vi "Argos.vi"(0 "PID 1 COM":refnum<visa-resource-name>="COM8", 1 "Setpoint\n START":bool, 2 "Write to File":bool, 3 "SP 1 input (°C)":dbl=20.0 min=0.0 max=1300.0, 4 "Intervall (s)":u32=1 max=600 format="%.2f", 5 "Write/\nRead":bool=TRUE, 6 "Delay (ms)":u32=500 min=100 max=600000, 7 "Auto Tune":bool, 9 "Standby":bool, 11 "Reset\nSTOPP":bool, 12 "ON":bool=TRUE caption="OFF", 13 "Get Values":bool, 15 "File Path":path) -> (8 "(°C)":dbl format="%#.3f", 14 "SP 1 is (°C)":dbl)   [LabVIEW 2010]
doc: "1. Verwendung\n\nDas Programm dient der Steuerung und Abfrage des Thermocontrollers I3252 und dem Auslesen von zwei VC 840 Messgeräten und einem Druckmessgerät Pfeiffer Single Gauge. \nDie Messgeräte werden Standardmäßig ausgelesen und erst nach Betätigung des Schalters \"Write to File\" in einer Textdatei abgespeichert. Das Eingabefeld \"Intervall\" legt den Abstand der Messpunkte fest.\nDer Setpoint für den Thermocontroller wird erst nach Betätigung des Tasters \"Setpoint START\" übernommen und angesteuert. Er wird ind den EEPROM des Gerätes geschrieben. Die Regelung kann mit Hilfe des Schalters \"Standby\" unterbrochen werden. Durch den Taster \"Reset STOPP\" kann der Setpoint aus dem EEPROM gelöscht werden.\nDie Eingabeflächen \"Constant\" und \"Thickness\" dienen der Berechnung des spezifischen Widerstands.\nDie Eingabeflächen \"User\" und \"Sample\" werden in den Header der Textdatei übernommen.\nDer Indikator \"File Path\" zeigt den aktuellen Speicherort der Textdatei an. Dieser wird nach ausschalten des Schalters \"Write to File\" gelöscht. Bei erneuten Schreiben muss ein neuer Speicherort gewählt werden. Bei Wahl desselben Speicherorts werden sämtliche bereits gespeicherte Daten gelöscht.\n\n\n2. Erläuterungen zum Blockdiagramm\n2.1 äußere Sequenz\nDie äußerte Sequenz besteht aus fünf Frames. Der erste dient der Initialisierung der Ports. Der zweite dient als Verzögerung um dem Programm genug Zeit zu geben die Ports zu öffnen. Jedoch senden die beiden VC 840 bereits Informationen an den Computer die in einem Puffer zwischengespeichert werden. Im dritten Frame wird dieser Puffer geleert. Somit kommt es zu keinem Framing Error. Desweiteren wird in diesem Frame die Startzeit der Messungen genommen. Im vierten Frame wird die eigentliche Messung und Verarbeitung der Daten durchgeführt. Die while-Schleife wird nur durch Auftreten eines Fehlers oder durch Betätigung des Stopbuttons auf dem Front Panel in der oberen linken Ecke unterbrochen. Im fünften und letzten Frame werden die Ports wieder geschlossen und beim Auftreten eines Fehlers wird das Programm automatisch gestoppt. Falls kein Fehler auftritt wird die Sequenz von vorne abgearbeitet.\n\n2.2 while-Schleife und innere Sequenz\n2.2.1 \"Event Structure\"\n2.2.1.1 Allgemein\nDer erste Frame beinhaltet ein \"Event Structure\". Dieser reagiert auf insgesamt elf verschiedene Ereignisse. Falls keines dieser Ereignisse auftreten sollte, warte die Struktur eine Millisekunde bevor die \"Event Structure\" verlassen wird. Die übrigen Ereignisse treten ein, wenn der entsprechende Kontroller eine Werteänderung erfährt.\n\n2.2.1.2 Event: Setpoint\nDieser Case besteht von außen nach innen aus einer Stacked Sequence, einer for-Loop und einer Flat Sequence die wiederum zwei \"Case Structures\" enthält. Als erstes wird bei dem Schalter \"Setpoint START\" der Blinkmodus aktiviert und bei dem Schalter \"Read Temperature\" deaktiviert. Danach folgt das eigentliche setzen des Temperatursollwerts. In der ersten Iteration wird dem Controller I3252 ein Schreibbefehl gesendet. Theoretisch kann der Setpoint in den RAM oder in den EEPROM geschrieben werden. Diese Auswahl erfolgt mit Hilfe des Schalters \"RAM\". Da das Schreiben in den RAM -Speicher aber aus diversen Gründen nicht erwünscht ist, wurde es nicht implementiert. Eine nachträgliche Implementierung ist aber leicht möglich, in dem die untere String-Konstante \"*P012\" durch \"*W012\" ersetzt wird. An diesem Befehl wird eine fünfstellige Hexadezimalzahl angehängt, die den Sollwert wiedergibt. Der Sollwert wird vorher mit zehn multipliziert, da das Komma standardmäßig nach der ersten Ziffer festgesetzt wurde (Bsp.: 800 wird gesendet um 80 einzustellen). Dieser Befehlsstrang wird an das Gerät mittels des SubVIs \"Comm_Interface\", auf welches später noch näher eingegangen wird, weitergegeben. Der durch das Gerät zurückgegebene String wird nicht verarbeitet.\nDie zweite Iteration dient dem Auslesen des eingestellten Sollwertes. Wahlweise kann der RAM- oder der EEPROM-Speicher ausgelesen werden. Die eigentliche Verarbeitung des Ausgabestrings erfolgt durch das SubVI \"Edit Setpoint\".\nDie Implementierung zur Einstellung des zweiten Setpoints erfolgt durch kopieren der ersten beiden Fälle und ersetzen der \"1\" im Befehf durch eine \"2\" (Bsp.: \"*P012\" zu \"*P022\"). Es darf aber nicht vergessen werden, dass dann ebenfalls die Anzahl der Iterationen angepasst werden muss.\nAls letztes wird der Blinkmodus des Schalters \"Setpoint START\" wieder deaktiviert.\n\n2.2.1.3 Event: Standby\nDieses Ereignis aktiviert bzw. deaktiviert als erstes den Blinckmodus des entsprechenden Schalters und sendet danach den Befehl zum aktivieren (\"*D03\") oder zum deaktivieren (\"*E03\") des Standbymodus an den Thermocontroller.\n\n2.2.1.4 Event: Set Command \nDer in das Feld \"Command shall be\" eingegebene Befehl wird an den Thermocontroller übermittlet. Die korrekte Form des Befehls ist im \"Communication Manuel\" nachzuschlagen. Das \"*\"-Zeichen wurde allerdings schon implementiert und muss somit nicht mit eingegeben werden.\n\n2.2.1.5 Event: Reset\nIn der ersten Iteration wird der Reset-Befehl an den Thermocontroller gesendet. In Folge wird der gesamte EEPROM-Speicher gelöscht. Deshalb wird in der zweiten Iteration der Setpoint aktualisiert. Dieser Befehl hat keinen Einfluss auf den RAM-Speicher. Die anschließende Wartezeit ist auf vier Sekunden festgesetzt und wurde empirisch ermittelt. Diese Zeit benötigt das Gerät um den Reset durchzuführen und für die Kommunikation wieder zur Verfügung zu stehen.\n\n2.2.1.6 Event: Auto Tune\nEs ist festgeschrieben, dass der Setpoint für die \"Auto Tune\"-Funktion wenigstens 20°C über der aktuellen Temperatur liegt. Deshalb wird zunächst der aktuelle Temperaturwert ausgelesen. Im zweiten Schritt werden zu diesem Wert zwanzig addiert und der Setpoint wird in den RAM-Speicher geschrieben. Das Schreiben in diesen Speicher ist nötig, da die \"Auto Tune\"-Funktion\" erst nach einem Reset startet. Im dritten Schritt wird der eigentliche Befehl für den \"Auto Tune\" gesendet (siehe dazu \"Communication Manuel\" S.27). Als vierte und letzte Iteration der for-Schleife folgt der bereits erwähnte Reset-Befehl. Der Temperatursollwert, der im RAM-Speicher eingetragen ist, muss zum Schluss wieder auf 0°C gesetzt werden. Die Zeit für die Ausführung des \"Auto Tune\"-Befehls wurde empirisch ermittelt und 45 s festgesetzt.\n\n2.2.1.7 Event: Write LOW/HI\nDieses Ereignis setzt die am Analogausgang anliegende Spannung fest. Normalerweise beträgt dieser Spannungswert 0-10 V. Das angeschlossene Netzteil verträgt aber maximal nur 2,3 V. Aus diesem Grund wird der \"%HIGH\" auf 23 gesetzt. Somit beträgt die maximal anliegende Spannung nur noch 23% von der maximal möglichen, d.h 2,3V. Ein niedrigerer Wert ist jederzeit möglich, genauso wie ein höherer für den Parameter \"%LOW\". Diese werden zunächst nacheinander in den RAM-Speicher geschrieben und anschließend wieder ausgelesen.\n\n2.2.1.8 Event: Set PID\nDie Werte für den PID-Regler können sowohl mit Hilfe der \"Auto Tune\"-Funktion, als auch manuell eingestellt werden. Es wird wiederum zwischen dem Schreiben in den RAM- und dem EEPROM-Speicher unterschieden. Zunächst werden die Werte für \"P\", \"I\" und \"D\", in dieser Reihenfolge, gesetzt und danach die aktuellen Werte ausgelesen.\n\n2.2.1.9 Event: Get Values\nDieses Ereignis hat zur Folge, dass die Werte für \"P\", \"I\", \"D\", \"%LOW\", \"%HIGH\" und des Setpoints wahlweise aus dem RAM- oder EEPROM-Speicher gelesen werden. Die aktuellen Werte werden nicht nur in die entsprechenden Anzeigefelder übernommen, sondern auch in die entsprechenden Eingabefelder, mit Ausnahme des Temperatursollwerts. \n\n2.2.1.10 Event: RAM\nPrinzipiell kann zwischen dem Schreiben in den RAM- oder EEPROM-Speicher des Thermocontrollers gewählt werden. Die entsprechende Schalterposition auf dem Frontpanel zeigt den aktuell verwendeten Speicher an. Die Anzeigewerte werden bei jedem Umschalten aktualisiert und sind im entsprechenden Speicher eingetragen. Die Implementierung ist identisch mit der des Ereignisses \"Get Values\". Es gilt zu beachten, dass die Werte für \"%LOW\" und \"%HIGH\" nur in den RAM-Speicher geschrieben werden können und somit auch nur aus diesem ausgelesen werden können.\n\n2.2.1.11 Event: Set Gauge to Zero\nMit Hilfe der SubVIs \"Get Pressure\" und \"Offset Display\" werden die Werte für den alten und den neuen Offset und der durch den zweiten Drucksensor ermittelt Druck ermittelt. \n\n2.2.1.12 Event: Write to File\nSollte der Schalter \"Write to File\" aktiviert werden, d.h. Schalterposition oben, so wird zunächst durch das SubVI \"Header\" ein Header für die unter \"File Path\" definierte Datei angelegt. Alle Werte, die bereits in der entsprechenden Datei stehen, werden dabei gelöscht.\n\n2.2.2 \"Timed Structures\"\nIm dritten Frame der inneren Sequenz werden die Werte für Zeitpunkt, Temperatur, Spannung, Strom und Druck ermittelt. Damit die Werte zum gleichen Zeitpunkt aufgenommen werden, werden \"Timed Sequences\" eingesetzt. Mit dem entsprechenden Schalter auf dem Front Panel unter dem Tab \"Settings\" kann gewählt werden, ob das entsprechende Gerät ausgelesen werden soll oder nicht. Die einzelnen Sequenzen werden parallel abgearbeitet, womit die Prozesszeit von diesem Frame durch der zeitintensivsten Sequenz abhängt. Dies ist in aller Regel das Auslesen der Temperatur, da ein \"Delay\" von 500 ms oder größer benötigt wird, um den Controller ordentlich ansprechen zu können.\nDie Systemzeit wird durch das SubVI \"System Time in Seconds\" in Sekunden umgerechnet und der in dem Parameter \"Starttime\" gespeicherte Wert wird abgezogen. Somit werden die Sekunden seit dem Start des Programms gezählt.\n\n2.2.3 restlichen Frames\nIm zweiten Frame wird das Intervall zwischen den einzelnen Messwerten festgelegt. Dabei wird der Wert des Parameters \"Delay\" abgezogen. Dieser Wert beträgt im Normalfall 500 ms und ist somit nicht vernachlääsigbar.\nDer Vierte Frame beinhaltet die Umrechnung des Temperatur-Strings in einen Temperaturwert durch das SubVI \"Edit Tmperature\", die Berechnung des spezifischen Widerstands durch das SubVI \"Resistivity Calculation\" und die Überprüfung des Druckwerts. Auch werden die neu gewonnen Werte in das entsprechende Shift-Register übernommen. Falls der Druckwert einen in dem Parameter \"Pressure Limit (mbar)\" festgelegten Grenzwert überschreiten sollte, wird der Thermocontroller automatisch in den Standby-Modus versetzt. Des Weiteren wird der Schalter \"Standby\" solange gesperrt, wie der Druck oberhalb des Grenzwertes liegt. Wenn der Druck wieder unter den Grenzwert gesunken ist, wird der Standby-Befehl nicht automatisch aufgehoben, sondern muss vom Benutzer durch Betätigung des entsprechenden Schalters gegeben werden.\nIm fünften Frame werden die Diagramme erstellt. Dabei wird jedes Mal von neuem das gesamte Shift-Register als Graph dargestellt. Weiterhin werden die Messwerte in ein 1D-Array geschrieben.\nDer sechste und letzte Frame beinhaltet den eigentlich Schreibvorgang der Messwerte in eine Textdatei und die Überprüfung ob ein Fehler vorliegt.\n\n2.3 SubVIs\n2.3.1 Allgemein\nDie SubVIs für die Messgeräte VC840 und das Druckmessgerät wurden aus anderen Quellen übernommen. \n\n2.3.2 \"Header\"\nIn den Header wird zunächst das aktuelle Datum und die aktuelle Zeit übernommen. Die ausgewählte Datei wird dabei überschrieben. Danach wird der Name des Benutzers und der Probe übernommen. Zum Schluss werden die Einheiten in einer Reihe, durch einen Tabulator getrennt, in den Header geschrieben.\n\n2.3.3 \"I3252 Comm Interface\"\nDieses VI stellt die Kommunikation mit dem Thermocontroller her und gibt den Ausgabe-String zurück.\n\n2.3.4 \"I3252 Edit Setpoint\"\nIm Ausgabe-String vom Thermocontroller ist an der vierten Stelle die Stelle des Dezimalpunktes verschlüsselt. Dieses Hexadezimalzahl wird herausgefiltert und an ein \"ENUM Controller\" übergeben. Dieser weist der Hexadezimalzahl eine Nummer zu, mit welcher ein Wert aus einem Array entnommen wird. Dieser Wert dient als Quotient. Der tatsächliche Wert kann somit errechnet werden.\n\n2.3.5 \"I3252 Edit Temperature\"\nDer Temperatur-String, der vom Thermocontroller zurückgegeben wird, wird in eine Dezimalzahl umgewandelt. Manchmal kommt es aus zu Dropouts, die durch dieses Programm herausgefiltert werden. Der letzte Wert wird dabei in einer \"Feedback Node\" gehalten unter der Annahme, dass sich der Temperaturwert nicht sprunghaft ändert.\n\n2.3.6 \"Resistivity Calculation\"\nDer spezifische Widerstand wird nach folgender Formel ausgerechnet. Dabei entspricht t der Dicke der Probe und C ist eine Konstante.\nrho=C*pi*t*U/(ln( 2)*I)\n\n2.3.7 \"System Time in Seconds\"\nZunächst wird die aktuelle Systemzeit ausgelesen. Danach wird diese in Stunden, Minuten und Sekunden aufgeteilt, alles in Sekunden umgerechnet und letztendlich addiert."
uses:
  <vilib>/Platform/TimedLoop/XDataNode/XDataNode.xnode
  <vilib>/Platform/TimedLoop/XDataNode/timing_clust.ctl
  <vilib>/Platform/TimedLoop/XDataNode/nitl_modes.ctl
  <vilib>/Platform/TimedLoop/XDataNode/wakeup.ctl
  <vilib>/Instr/_visa.llb/VISA Configure Serial Port (Instr).vi
  <vilib>/Platform/TimedLoop/scheduler/LVUserAPI/_suppVIs/Create_1kHz_TSource.vi
  <vilib>/Utility/file.llb/Write To Spreadsheet File (DBL).vi
  <vilib>/Platform/TimedLoop/XDataNode/XDNodeRunTimeDep.lvlib
  Pfeiffer TPG261+262 Single+Dual Gauge/Dual Gauge.lvlib
panel:
  out "error out":errorcluster
  out "appended array":dbl[](array[numeric])
  in  "Tab Control":T1(tab)
  in  "Thickness (nm)":dbl min=0.0
  in  "4PP constant":dbl min=0.0 max=5.0
  in  "Sample":string
  in  "User":string
  out "Sample holder (Type-K Thermocouple)":cluster{dbl[], dbl[]}(graph)
  out "current time (s)":dbl
  out "data logger intervall (s)":dbl
  out "loop time (s)":ext
  in  "stop":bool
  out "Main Chamber (PG-1)":cluster{dbl[], dbl[]}(graph)
  out "Pressure Gauge 1#1":dbl format="%#_4e"
  out "Loadlock (PG-3)":cluster{dbl[], dbl[]}(graph)
  out "Pressure Gauge 1#2":dbl format="%#_3e"
  out "Pressure Gauge 2#1":dbl format="%#_3e"
  out "Pressure OpenPort":cluster{dbl[], dbl[]}(graph)
  out "Pressure Gauge 2#2":dbl caption="current"
  out "Pirani (VVP1 Scroll)":cluster{dbl[], dbl[]}(graph)
  out "status 2":bool caption="Status"
  out "code 2":i32 caption="Code"
  out "code":i32 caption="Code"
  out "status":bool caption="Status"
  in  "Set Gauge to Zero":bool
  out "Status Gauge 1#2":i32(ring) items=["data OK", "underrange", "overrange", "sensor error", "sensor off", "no sensor", "ID error"]
  out "Pressure Gauge 1#2":dbl format="%.3e"
  out "Pressure Gauge 1#1":dbl format="%.3e"
  out "Status Gauge 1#1":i32(ring) items=["data OK", "underrange", "overrange", "sensor error", "sensor off", "no sensor", "ID error"]
  in  "TPG 1 COM":refnum<visa-resource-name>="COM5"
  in  "Pressure Limit (mbar)":dbl=1.0 min=0.0 max=1100.0
  out "Current Offset (mbar)":dbl
  in  "ON (TPG 2)":bool caption="OFF"
  in  "ON (TPG 1)":bool=TRUE caption="OFF"
  in  "ON":bool caption="OFF"
  in  "VC 840 2":refnum<visa-resource-name>="COM9"
  out "Reading 2":dbl format="%_4f"
  out "Mode 2":enum16{"?", "Diode", "Beep", "DC", "AC"}(ring)
  out "Unit 2":string
  in  "VC 840 1":refnum<visa-resource-name>="COM9"
  out "Reading 1":dbl format="%_4f"
  out "Mode 1":enum16{"?", "Diode", "Beep", "DC", "AC"}(ring)
  out "Unit 1":string
  out "Status 1":T2
  out "Status 2":T2
  in  "ON":bool caption="OFF"
  out "% HIGH Istwert":u32
  out "% LOW Istwert":u32
  in  "% High Sollwert":u32=23 max=24
  in  "% LOW Sollwert":u32 max=25
  in  "RAM":bool=TRUE caption="EEPROM"
  out "D (Rate) IstWert":u32
  out "I ( Reset1) Istwert":u32
  out "P (PB1) Istwert":u32 caption="actual value"
  in  "D (Rate) Sollwert":u32 max=3999
  in  "I ( Reset1) Sollwert":u32 max=3999
  in  "P (PB1) Sollwert":u32 caption="set value" max=9999
  in  "Set Command":bool
  in  "Set PID":bool
  in  "Write LOW/HI":bool
  in  "Flow Control":u16(ring) items=["None"=0, "XON/XOFF"=1, "RTS/CTS"=2, "DTR/DSR"=4]
  in  "Stop Bits":u16(ring)=10 items=["1.0"=10, "1.5"=15, "2.0"=20]
  in  "Parity":u16(ring)=1 items=["None", "Odd", "Even", "Mark", "Space"]
  in  "Data Bits":u16=7 min=5 max=8 step=1
  in  "Baud Rate":u32=9600
  out "Command output":string
  in  "Command input":string
  in  "TPG 2 COM":refnum<visa-resource-name>="COM6"
  out "Pressure Gauge 2#2":dbl format="%.3e"
  out "Pressure Gauge 2#1":dbl format="%.3e"
  out "Status Gauge 2#2":i32(ring) items=["data OK", "underrange", "overrange", "sensor error", "sensor off", "no sensor", "ID error"]
  out "Status Gauge 2#1":i32(ring) items=["data OK", "underrange", "overrange", "sensor error", "sensor off", "no sensor", "ID error"]
  in  "VISA resource name":refnum<visa-resource-name>="COM1"
  in  "baud rate (9600)":u32=9600
  in  "data bits (8)":u16=8 min=5 max=8 step=1
  in  "parity (0:none)":enum16{"None", "Odd", "Even", "Mark", "Space"}(ring)
  in  "stop bits (10: 1 bit)":u16(ring)=10 items=["1.0"=10, "1.5"=15, "2.0"=20]
  in  "flow control (0:none)":u16(ring) items=["None", "XON/XOFF", "RTS/CTS", "XON/XOFF & RTS/CTS", "DTR/DSR", "XON/XOFF & DTR/DSR"]
  out "command to Keithley":string
  in  "output current setpoint (A)":dbl caption="setpoint" max=9999.0 format="%.4f"
  out "Bytes at Port":u32
  out "actual value":string
  in  "Set Output Current":bool
  out "Bytes at Port 3":u32
  out "read buffer 2":string
  in  "RUN Keithley Measurement":bool
  in  "Keithley delay (ms)":u32=500
  out "Current":cluster{dbl[], dbl[]}(graph)
  out "Voltage":cluster{dbl[], dbl[]}(graph)
  out "Voltage (V)":dbl format="%.4e"
  out "Current (A)":dbl format="%.4e"
  out "Resistivity":cluster{dbl[], dbl[]}(graph)
  out "Resistivity (Ohm*cm)":dbl format="%.3e"
  # "set \nvalue"
  # "actual \nvalue"
  # "T (°C)"
  # "mbar"
  # "mbar"
  # "mbar"
  # "mbar"
  # "Pressure Measurement \n(Pfeiffer TPG261)"
  # "PID Controller (Omega Newport i3252)"
  # "limit (mbar)"
  # "Multimeter\n#1 (VC 840)"
  # "Multimeter\n#2 (VC 840)"
  # "P"
  # "I"
  # "D"
  # "% Low"
  # "% High"
  # "Authors:  Daniel Schuster (sir-dan@web.de)\n                 Steffen Cornelius (s.cornelius@hzdr.de)\n                 Nico Spahn (x)\n\n                 premade SubVIs for readout of Pfeiffer gauge and VC840 Multimeters were used\n                 SubVI \"I3252_Comm_Interface\" is based on a modified Labview example\n\nRelease:  v1.0    \n\nVersion History:\n\nv1.1  -    28.06.2011\n             - Format des Files geändert von %.3f auf %g\n             - maximale Eingabewerte für PID begrenzt\nv1.2  -    12.07.2011\n             - Anzeige p,rho, U, V auf Scientific geändert\n             - y-Achse p,rho auf Log geändert\n             - numerische Zeitanzeige hinzugefügt\n             - 4PP Constant: pi/ln(2)=4,532 set as the default value\nv1.3  -    25.07.2011\n             - Zeitvariable auf EXT geändert, um Sprünge in Diagrammen loszuwerden\nv1.4  -   27.07.2011\n             - ALLE Variablen auf DBL zurückgesetzt wegen Formatierungsproblem im File\n             - Zeitberechnung neu gemacht (Tick count differenzen) -> Zeitsprünge korrigiert ?\n             - Delay/Intervall überarbeitet\nv1.5  -   05.12.2012\n                - Austausch der alten Pfeifer SubvIs durch neue -> nun alle 4 Kanäle des DualGauge\n                                                                                                         Controllers gleichzeitig auslesbar\n                - neue Pfeiffer SubVIs verwendet in Druckwertauslesung und Offset Berechnung des Baratron\n                  Druckes (COM5 Sensor1)\n                - Neuarragement des GUI -> FullRange und Baratron neben Temperatur auf Haupseite zu sehen\n                                                                   Pirani und OpenPort auf Meas.2 zu sehen\n                                                                   Diagnose Seite umfasst nun auch Widerstandsdiagramm\n                - Änderungen der Settingseite -> nun alle 4 Drucksensoren mit aktuellem Messwert und Gerätestatus\n                                                                           zu sehen\n                - The readout of the PID-Temperature Controller and the VC840 Multimeters was not modified\nv1.73  -  18.10.2013\n                - Layout Änderungen\nv.1.8   -  19.01.2014\n                - Änderung Layout Settings Tab\n                - Trennung der beiden TPG Dual Gauge Controls\n                -"
  # "Version 1.73    - last change 18.10.2013"
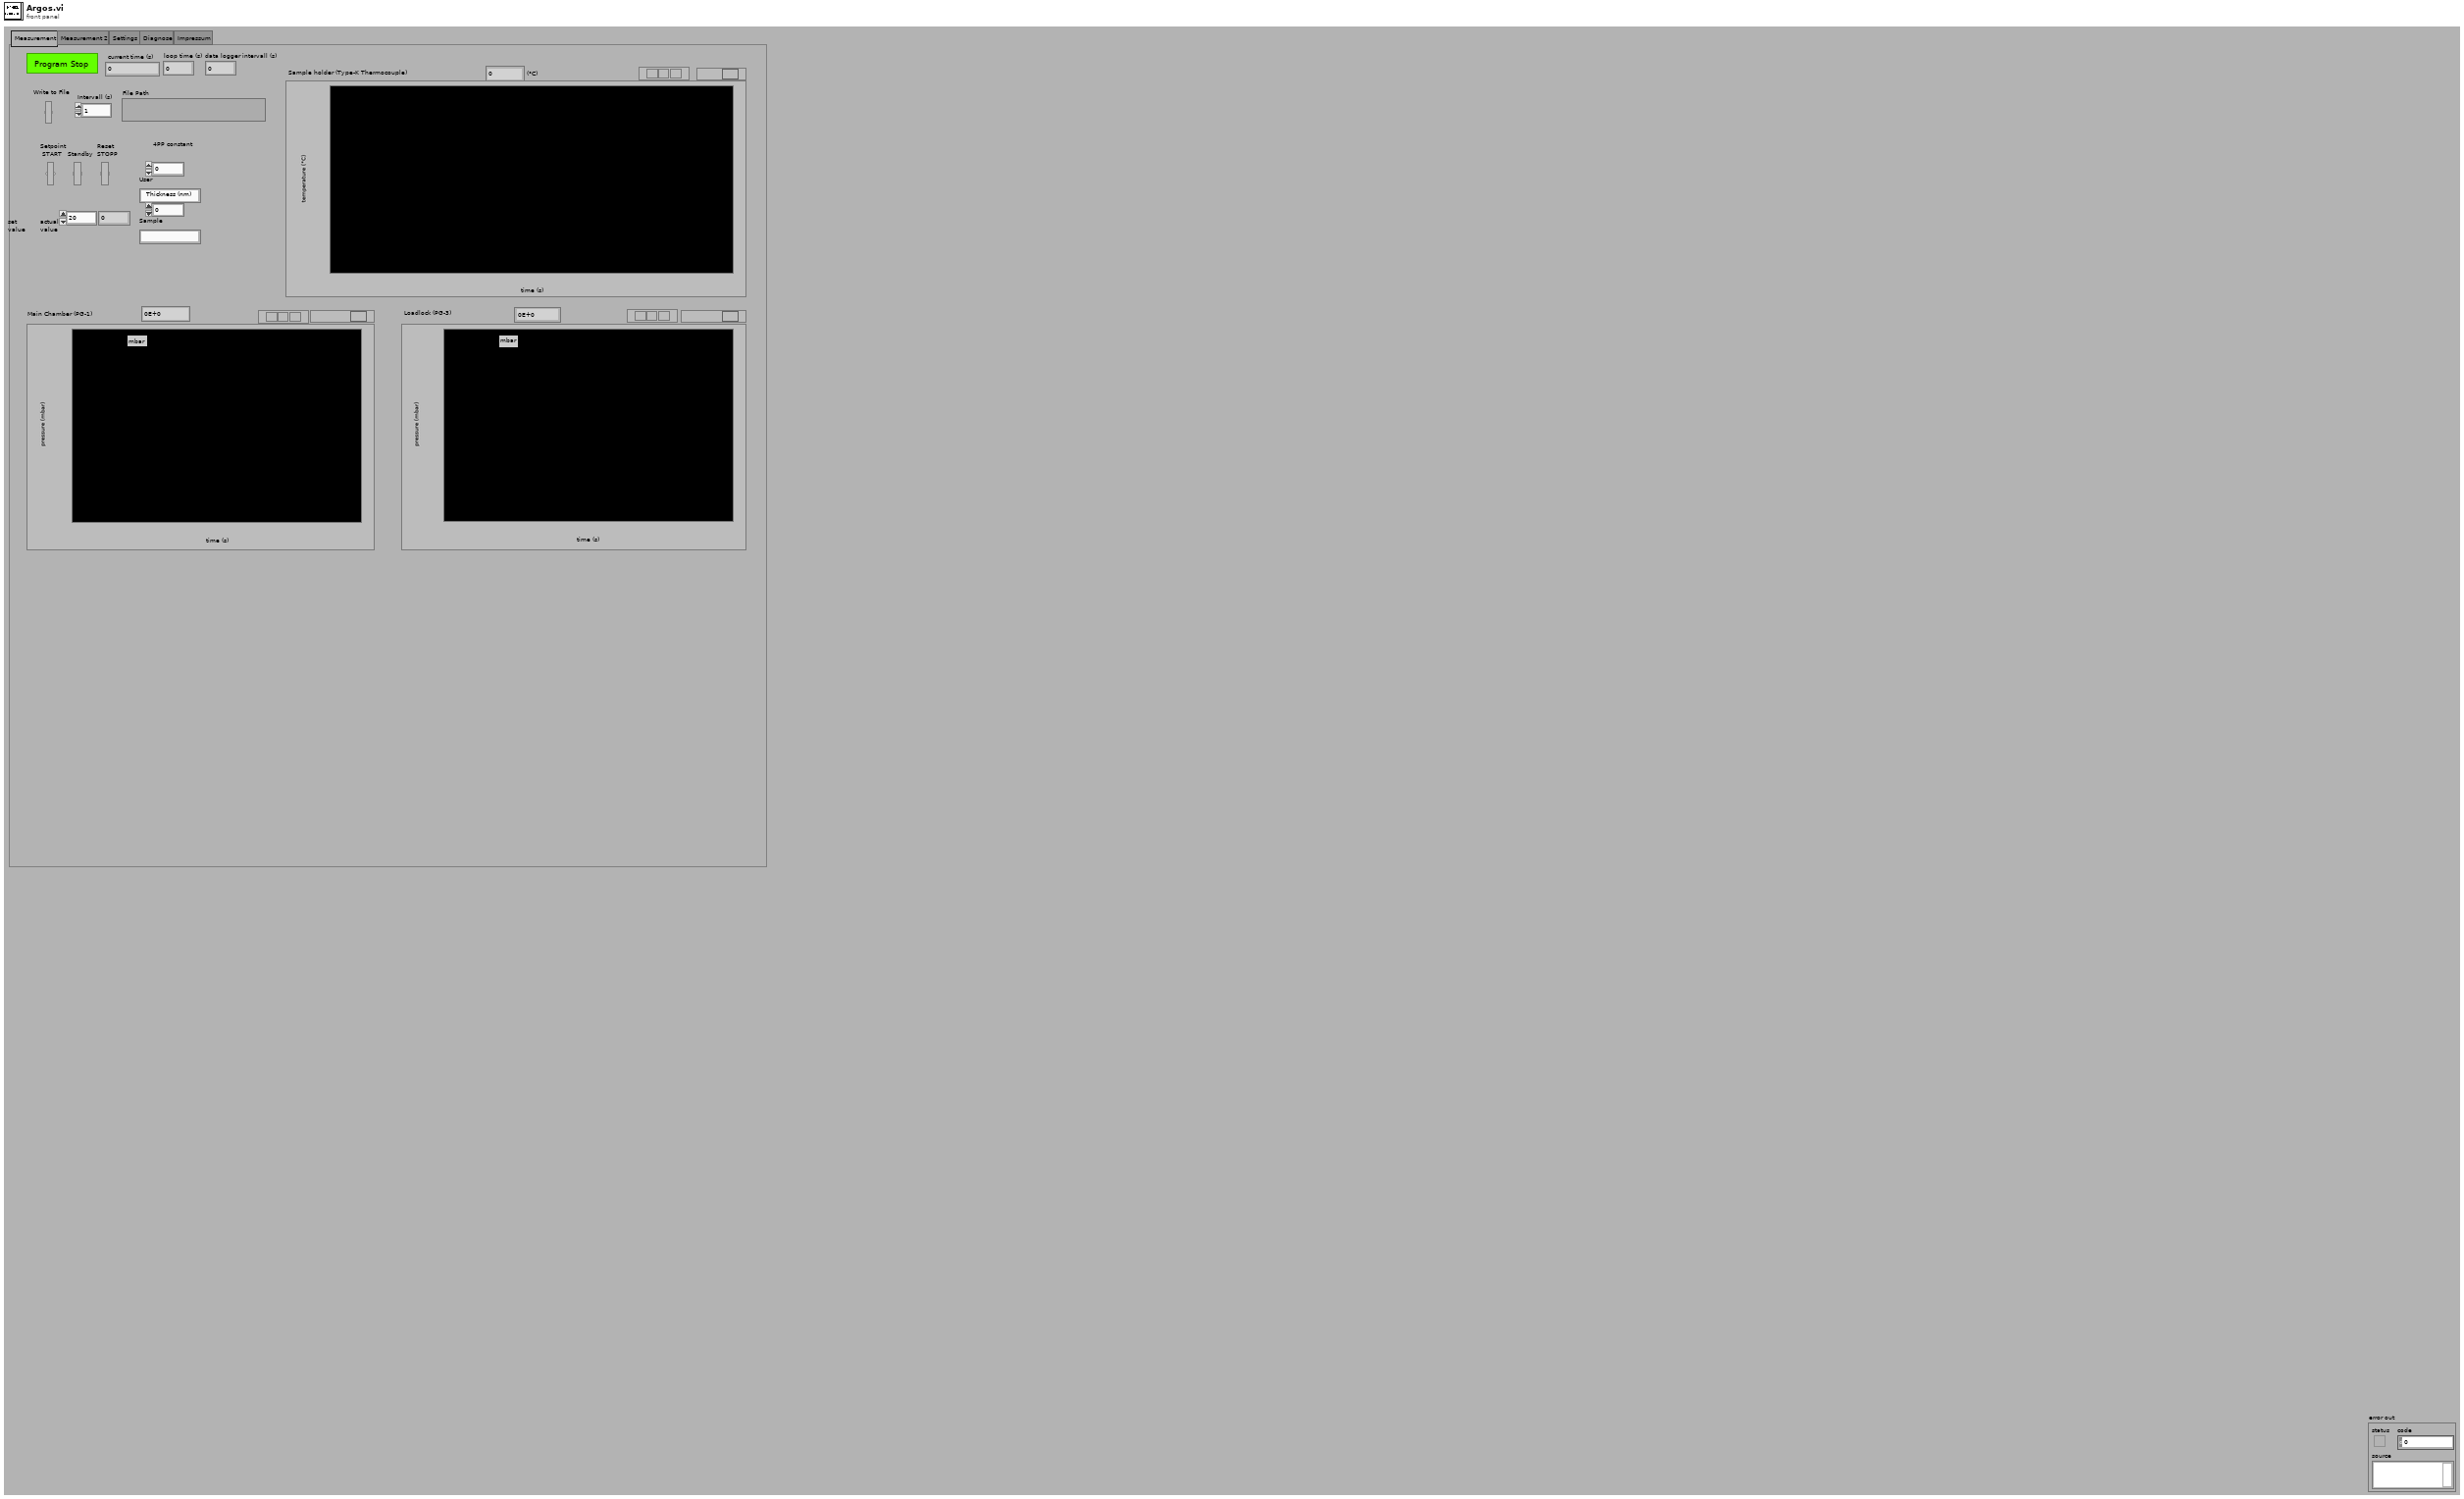
[diagram p1: front panel]
types:
  T1 = enum32{"Measurement", "Measurement 2", "Settings", "Diagnose", "Impressum"}
  T2 = cluster{"Low Bat":bool, "Auto":bool, "Delta":bool, "Hold":bool, "RS232":bool}
  T3 = typedef "XDNodeRunTimeDep.lvlib/timing_clust.ctl" = cluster{"Expected End [f-1]":u64, "Actual End [f-1]":u64, "Finished Late? [f-1]":bool, "Expected End [i-1]":u64, "Actual End [i-1]":u64, "Finished Late? [i-1]":bool, "Expected Start [i]":u64, "Actual Start [i]":u64, "Expected Start [f]":u64, "Actual Start [f]":u64, "Source Name":string, "Structure Name":string, "Period":i64, "Deadline":i64, "Offset":i64, "Start":i64, "Priority":i32, "Timeout":i32, "Mode":T4, "Wakeup Reason":T5, "Error":errorcluster, "Source Type":string, "Secondary Source Type":string, "Global End Time":u64, "Global Start Time":u64, "Frame Duration":u64, "Iteration Duration":u64, "Assigned CPU":i32, "I/O Scan Engine Mode":u32}
  T4 = typedef "XDNodeRunTimeDep.lvlib/nitl_modes.ctl" = enum32{"No Change", "Process missed periods, maintain original phase", "Discard missed periods, maintain original phase", "Process missed periods, ignore original phase", "Discard missed periods, ignore original phase"}
  T5 = typedef "XDNodeRunTimeDep.lvlib/wakeup.ctl" = enum32{"Normal", "Aborted", "Asynchronous wakeup", "Timing source error", "Timed loop error", "Timeout"}
  T6 = enum8{"Enabled", "Disabled", "Disabled and Grayed Out"}
  T7 = cluster{"VISA resource name out":refnum<visa-resource-name>, "error out":errorcluster, "Delay (ms)":u32, "Write/\nRead":bool}
  T8 = cluster{"TPG 2 COM":refnum<visa-resource-name>, "error out":errorcluster}
  T9 = cluster{"COM out":refnum<visa-resource-name>, "Cluster (Ausgang)":errorcluster}
  T10 = cluster{"Pressure Gauge#1":dbl, "Pressure Gauge#2":dbl}
  T11 = cluster{"TPG 1 COM":refnum<visa-resource-name>, "error out":errorcluster}
  T12 = cluster{"COM out":refnum<visa-resource-name>, "error out":errorcluster, "COM out":refnum<visa-resource-name>, "error out":errorcluster}
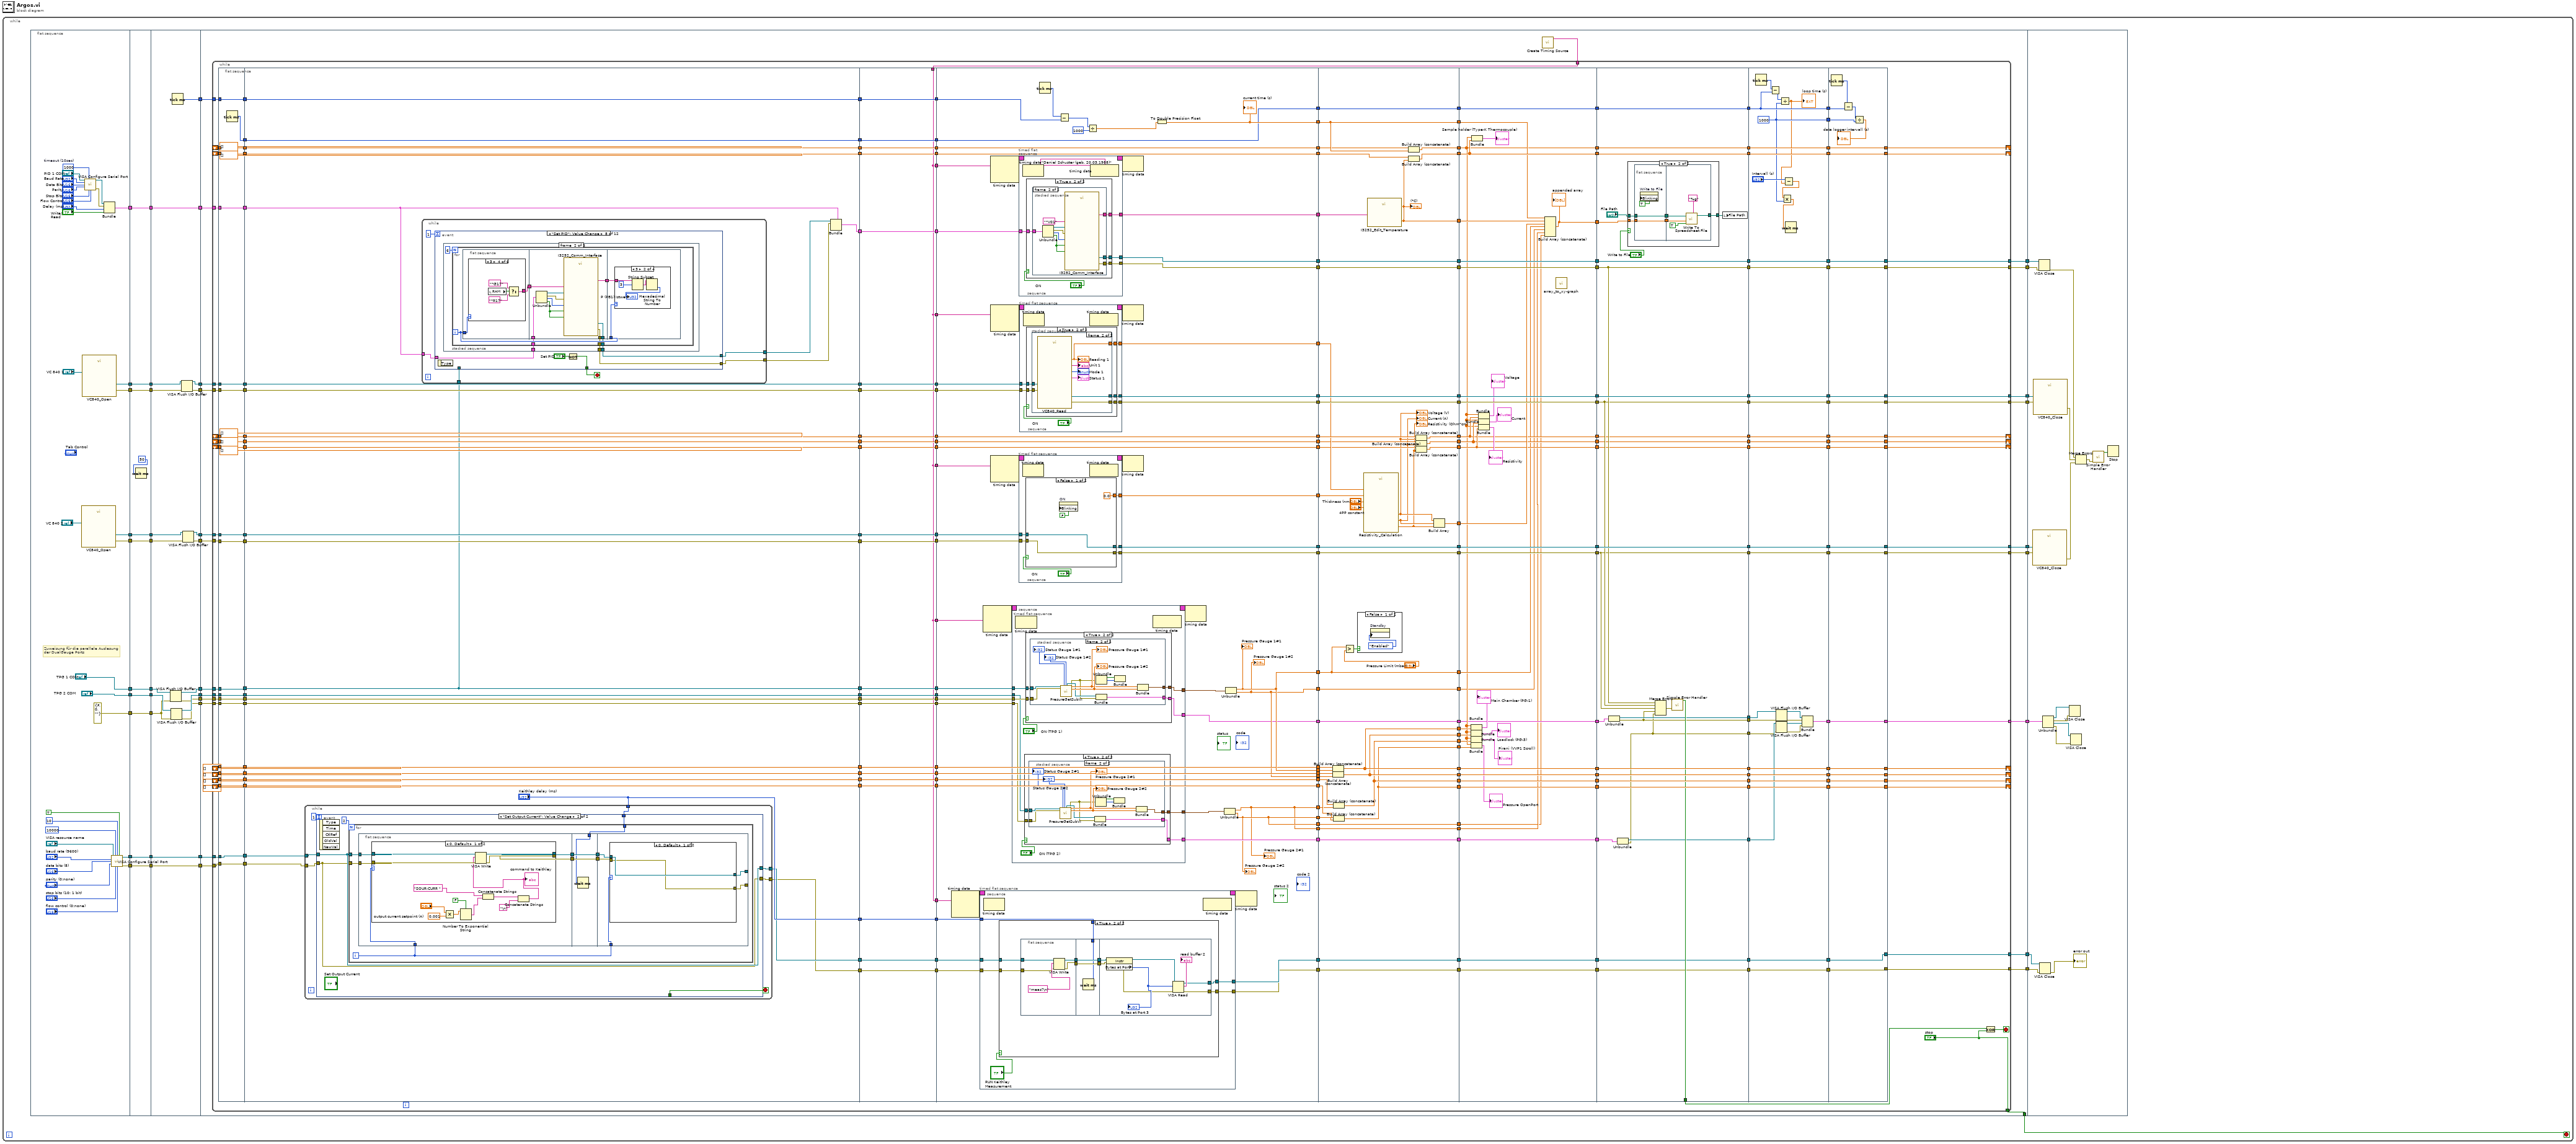
[diagram p0: block diagram]
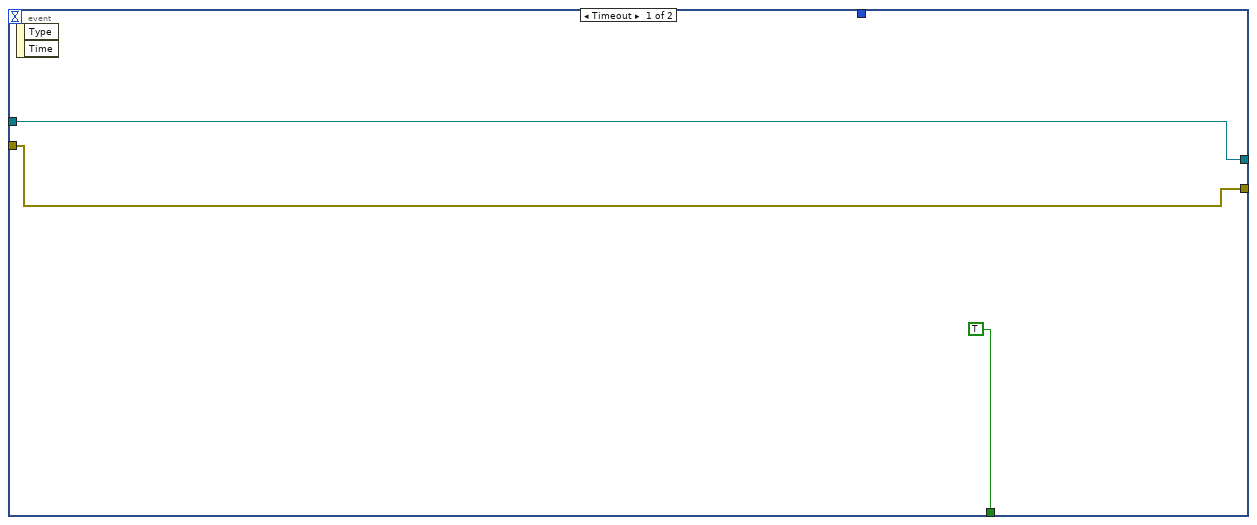
[diagram p2: hidden frame]
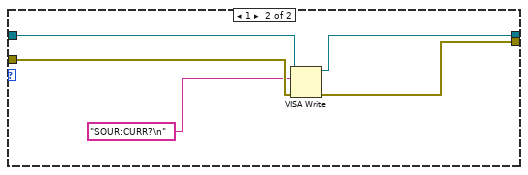
[diagram p3: hidden frame]
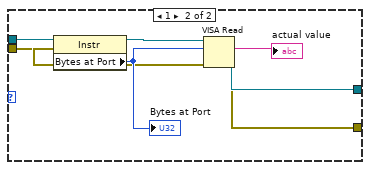
[diagram p4: hidden frame]
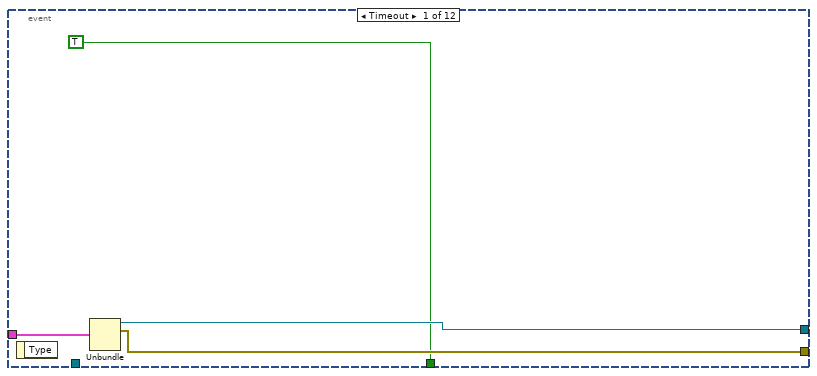
[diagram p5: hidden frame]
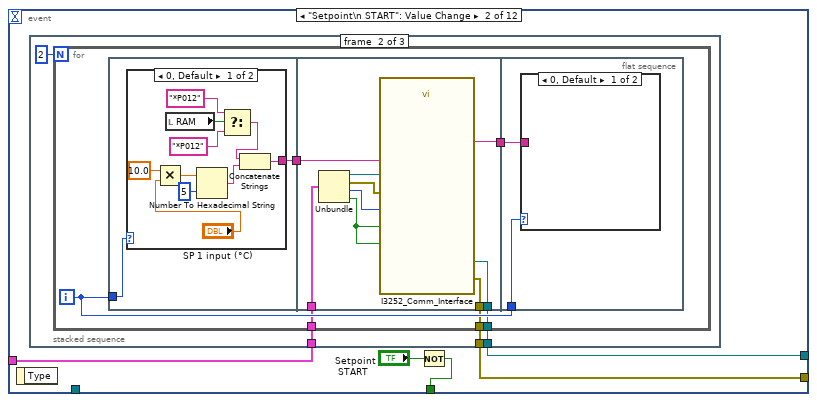
[diagram p6: hidden frame]
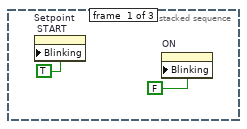
[diagram p7: hidden frame]
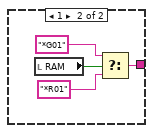
[diagram p8: hidden frame]
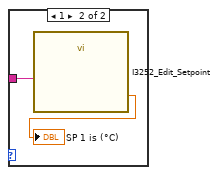
[diagram p9: hidden frame]
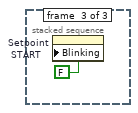
[diagram p10: hidden frame]
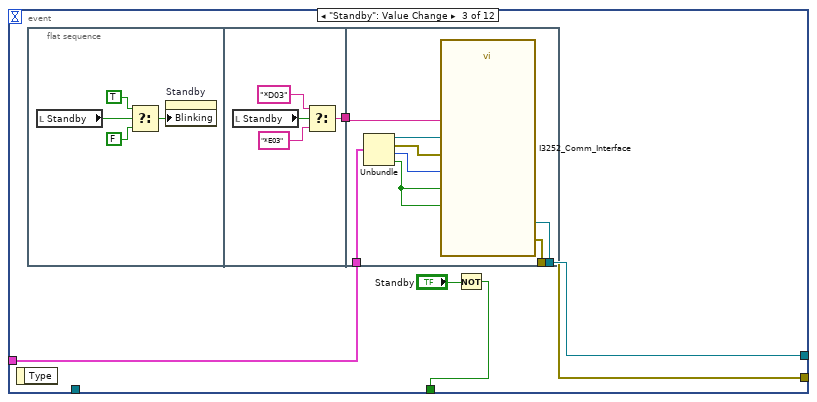
[diagram p11: hidden frame]
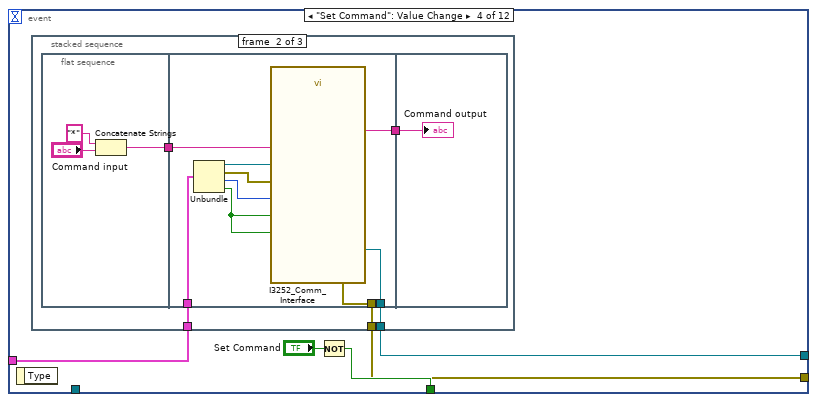
[diagram p12: hidden frame]
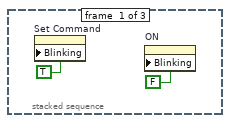
[diagram p13: hidden frame]
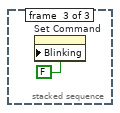
[diagram p14: hidden frame]
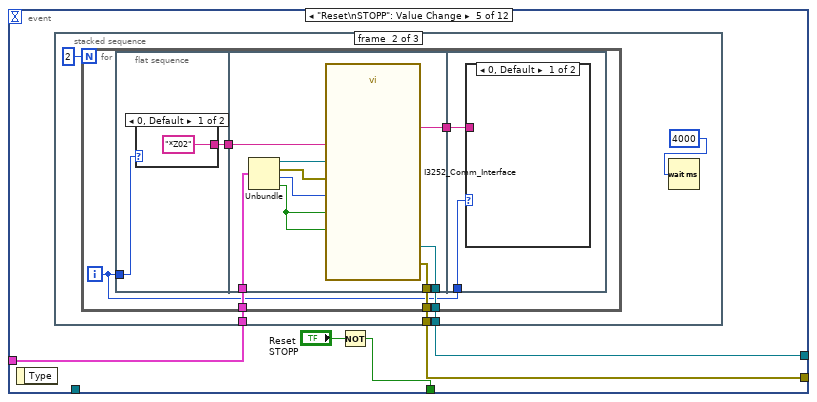
[diagram p15: hidden frame]
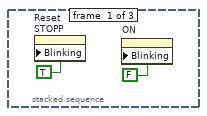
[diagram p16: hidden frame]
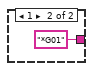
[diagram p17: hidden frame]
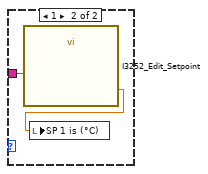
[diagram p18: hidden frame]
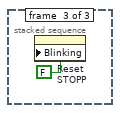
[diagram p19: hidden frame]
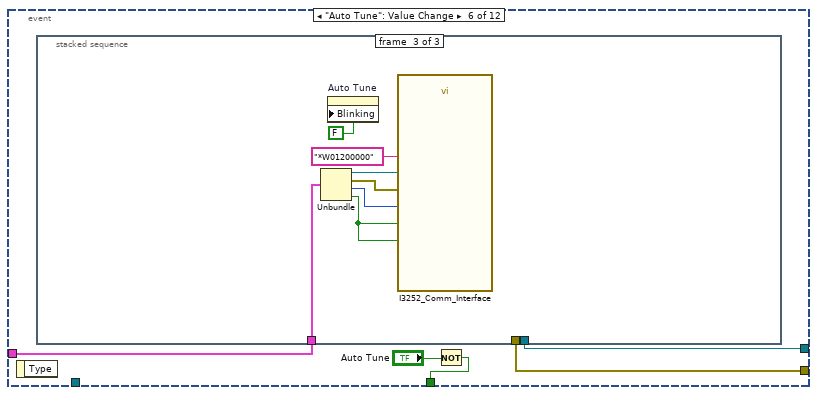
[diagram p20: hidden frame]
diagram:
  n1 = while {
    stop <- w14 stop-if-true
    n2 = flat-sequence {
      tunnel: [w73] -> w42
      tunnel: [w74] -> w41
      tunnel: [w59] -> w40
      tunnel: [w72] -> w39
      tunnel: [w71] -> w38
      tunnel: ["TPG 1 COM"] -> w37
      tunnel: ["TPG 2 COM"] -> w36
      tunnel: [errorcluster {"status"=FALSE, "code"=0, "source"=""} ("Fehler (Eingang)")] -> w11
      tunnel: [w44] -> w4
      tunnel: [w43] -> w3
      tunnel: w42 -> [w85]
      tunnel: [w85] -> w35
      tunnel: w41 -> [w84]
      tunnel: [w84] -> w34
      tunnel: w40 -> [w83]
      tunnel: [w83] -> w33
      tunnel: w39 -> [w82]
      tunnel: [w82] -> w32
      tunnel: w38 -> [w81]
      tunnel: [w81] -> w31
      tunnel: [w79] -> w30
      tunnel: w37 -> [w79]
      tunnel: [w78] -> w29
      tunnel: w36 -> [w78]
      tunnel: [w77] -> w12
      tunnel: w11 -> [w77]
      tunnel: [w76] -> w5
      tunnel: w4 -> [w76]
      tunnel: w3 -> [w75]
      tunnel: [w75] -> w2
      tunnel: w35 -> [w98]
      tunnel: [w97] -> w28
      tunnel: w34 -> [w99]
      tunnel: [w96] -> w27
      tunnel: w33 -> [w104]
      tunnel: [w104] -> w26
      tunnel: w32 -> [w101]
      tunnel: [w102] -> w25
      tunnel: w31 -> [w100]
      tunnel: [w103] -> w24
      tunnel: [w95] -> w23
      tunnel: [w93] -> w22
      tunnel: w30 -> [w94]
      tunnel: [w92] -> w21
      tunnel: w29 -> [w91]
      tunnel: w12 -> [w90]
      tunnel: [w89] -> w10
      tunnel: [w88] -> w9
      tunnel: [w87] -> w6
      tunnel: w5 -> [w87]
      tunnel: w2 -> [w86]
      tunnel: [w86] -> w1
      tunnel: w28 -> [w136]
      tunnel: w27 -> [w135]
      tunnel: w26 -> [w134]
      tunnel: w25 -> [w132]
      tunnel: w24 -> [w131]
      tunnel: [w130] -> w20
      tunnel: [w129] -> w19
      tunnel: [w128] -> w18
      tunnel: [w127] -> w17
      tunnel: [w126] -> w16
      tunnel: [w125] -> w15
      tunnel: w23 -> [w119]
      tunnel: w22 -> [w118]
      tunnel: w21 -> [w117]
      tunnel: [w112] -> w14
      tunnel: [w111] -> w13
      tunnel: w10 -> [w110]
      tunnel: w9 -> [w109]
      tunnel: [w108] -> w8
      tunnel: [w107] -> w7
      tunnel: w6 -> [w106]
      tunnel: w1 -> [w105]
      tunnel: w20 -> [w1503]
      tunnel: w19 -> [w1502]
      tunnel: w18 -> [w1505]
      tunnel: w17 -> [w1504]
      tunnel: w16 -> [w1507]
      tunnel: w15 -> [w1506]
      tunnel: w13 -> [w1500]
      tunnel: w8 -> [w1494]
      tunnel: w7 -> [w1493]
      frame #0 {
        w60 = u32 1000  # timeout (10sec)
        # "Zuweisung für die parallele Auslesung\nder DualGauge Ports"
        n3 = call "VC840_Open.vi"("VISA resource name"="VC 840 2") -> ("error out"=w71:errorcluster, "VISA resource name out"=w72:refnum<visa-resource-name>)  [unwired: 1 in, 8 out]
        n4 = call "VC840_Open.vi"("VISA resource name"="VC 840 1") -> ("error out"=w74:errorcluster, "VISA resource name out"=w73:refnum<visa-resource-name>)  [unwired: 1 in, 8 out]
        n5 = call-poly "VISA Configure Serial Port"("VISA resource name"="PID 1 COM", "timeout (10sec)"=w60, "baud rate (9600)"="Baud Rate", "data bits (8)"="Data Bits", "parity (0:none)"="Parity", "stop bits (10: 1 bit)"="Stop Bits", "flow control (0:none)"="Flow Control") -> ("VISA resource name out"=w69:refnum<visa-resource-name>, "error out"=w70:errorcluster)  [unwired: 2 in, 5 out]
        n6 = Bundle("VISA resource name out"=w69, "error out"=w70, "Delay (ms)"="Delay (ms)", "Write/\nRead"="Write/\nRead") -> (w59:T7)  [unwired: 1 in]
        n7 = call-poly "VISA Configure Serial Port"("VISA resource name"="VISA resource name", "timeout (10sec)"=u32 10000, "termination char\n(0xA = '\\n' = LF)"=u8 10 ("termination char\n(0xA = '\\n' = LF)"), "Enable Termination\nChar (T)"=TRUE ("Enable Termination\nChar (T)"), "baud rate (9600)"="baud rate (9600)", "data bits (8)"="data bits (8)", "parity (0:none)"="parity (0:none)", "stop bits (10: 1 bit)"="stop bits (10: 1 bit)", "flow control (0:none)"="flow control (0:none)") -> ("VISA resource name out"=w44:refnum<visa-resource-name>, "error out"=w43:errorcluster)  [unwired: 5 in]
      }
      frame #1 {
        n8 = Wait (ms)(milliseconds to wait=u32 50) -> ()  [unwired: 1 out]
      }
      frame #2 {
        n9 = VISA Flush I/O Buffer(VISA resource name=w94, error in (no error)=w90) -> (VISA resource name out=w93:refnum<visa-resource-name>, error out=w89:errorcluster)  [unwired: 1 in]
        n10 = VISA Flush I/O Buffer(VISA resource name=w91, error in (no error)=w90) -> (VISA resource name out=w92:refnum<visa-resource-name>, error out=w88:errorcluster)  [unwired: 1 in]
        n11 = Tick Count (ms)() -> (millisecond timer value=w95:u32)
        n12 = VISA Flush I/O Buffer(VISA resource name=w98, error in (no error)=w99) -> (VISA resource name out=w97:refnum<visa-resource-name>, error out=w96:errorcluster)  [unwired: 1 in]
        n13 = VISA Flush I/O Buffer(VISA resource name=w101, error in (no error)=w100) -> (VISA resource name out=w102:refnum<visa-resource-name>, error out=w103:errorcluster)  [unwired: 1 in]
      }
      frame #3 {
        n14 = call-poly <vilib>:"Create Timing Source.vi"() -> ("name (out)"=w133:string)  [unwired: 10 in, 1 out]
        n15 = while {
          tunnel: w136 -> [w378]
          tunnel: w135 -> [w377]
          tunnel: w134 -> [w376]
          tunnel: w133 -> [w369]
          tunnel: w132 -> [w362]
          tunnel: w131 -> [w361]
          tunnel: [w357] -> w130
          tunnel: [w356] -> w129
          tunnel: [w354] -> w128
          tunnel: [w352] -> w127
          tunnel: [w350] -> w126
          tunnel: [w348] -> w125
          shift-right: [w321] -> _
          shift-left: dbl[] [] -> [w326]
          shift-right: [w299] -> _
          shift-left: dbl[] [] -> [w334]
          shift-right: [w323] -> _
          shift-left: dbl[] [] -> [w330]
          shift-right: [w296] -> _
          shift-left: dbl[] [] -> [w333]
          shift-right: [w293] -> _
          shift-left: dbl[] [] -> [w332]
          tunnel: w119 -> [w287]
          tunnel: w118 -> [w243]
          tunnel: w117 -> [w239]
          shift-right: [w197] -> _
          shift-left: dbl[] [] -> [w227]
          shift-right: [w195] -> _
          shift-left: dbl[] [] -> [w225]
          shift-right: [w193] -> _
          shift-left: dbl[] [] -> [w223]
          shift-right: [w191] -> _
          shift-left: dbl[] [] -> [w221]
          tunnel: ["stop"] -> w112
          tunnel: [w185] -> w111
          tunnel: w110 -> [w180]
          tunnel: w109 -> [w178]
          tunnel: [w159] -> w108
          tunnel: [w149] -> w107
          tunnel: w106 -> [w146]
          tunnel: w105 -> [w143]
          stop <- w184 stop-if-true
          n16 = flat-sequence {
            tunnel: w287 -> [w390]
            tunnel: w326 -> [w391]
            tunnel: w330 -> [w392]
            tunnel: w332 -> [w393]
            tunnel: w333 -> [w394]
            tunnel: w334 -> [w395]
            tunnel: w361 -> [w396]
            tunnel: w362 -> [w397]
            tunnel: w376 -> [w398]
            tunnel: w377 -> [w399]
            tunnel: w378 -> [w400]
            tunnel: [w400] -> w286
            tunnel: [w399] -> w285
            tunnel: [w398] -> w284
            tunnel: [w397] -> w283
            tunnel: [w396] -> w282
            tunnel: [w395] -> w281
            tunnel: [w394] -> w280
            tunnel: [w393] -> w279
            tunnel: [w392] -> w278
            tunnel: [w391] -> w277
            tunnel: [w390] -> w276
            tunnel: [w389] -> w258
            tunnel: [w388] -> w244
            tunnel: w243 -> [w388]
            tunnel: [w387] -> w240
            tunnel: w239 -> [w387]
            tunnel: [w386] -> w228
            tunnel: w227 -> [w386]
            tunnel: [w385] -> w226
            tunnel: w225 -> [w385]
            tunnel: [w384] -> w224
            tunnel: w223 -> [w384]
            tunnel: [w383] -> w222
            tunnel: w221 -> [w383]
            tunnel: [w382] -> w181
            tunnel: w180 -> [w382]
            tunnel: [w381] -> w179
            tunnel: w178 -> [w381]
            tunnel: w146 -> [w380]
            tunnel: [w380] -> w145
            tunnel: w143 -> [w379]
            tunnel: [w379] -> w144
            tunnel: [w428] -> w375
            tunnel: [w427] -> w373
            tunnel: [w423] -> w371
            tunnel: [w422] -> w366
            tunnel: [w421] -> w364
            tunnel: [w420] -> w331
            tunnel: [w419] -> w327
            tunnel: [w418] -> w307
            tunnel: [w417] -> w304
            tunnel: [w416] -> w302
            tunnel: [w415] -> w288
            tunnel: w286 -> [w428]
            tunnel: w285 -> [w427]
            tunnel: w284 -> [w426]
            tunnel: w283 -> [w422]
            tunnel: w282 -> [w421]
            tunnel: w281 -> [w418]
            tunnel: w280 -> [w417]
            tunnel: w279 -> [w416]
            tunnel: w278 -> [w420]
            tunnel: w277 -> [w419]
            tunnel: w276 -> [w415]
            tunnel: [w414] -> w259
            tunnel: w258 -> [w414]
            tunnel: w244 -> [w412]
            tunnel: [w412] -> w241
            tunnel: w240 -> [w413]
            tunnel: [w413] -> w237
            tunnel: w228 -> [w411]
            tunnel: w226 -> [w410]
            tunnel: w224 -> [w409]
            tunnel: w222 -> [w408]
            tunnel: [w411] -> w220
            tunnel: [w410] -> w216
            tunnel: [w409] -> w213
            tunnel: [w408] -> w212
            tunnel: w181 -> [w407]
            tunnel: w179 -> [w406]
            tunnel: [w407] -> w176
            tunnel: [w406] -> w174
            tunnel: w145 -> [w405]
            tunnel: w144 -> [w404]
            tunnel: ["Keithley delay (ms)"] -> w142
            tunnel: [w402] -> w140
            tunnel: [w401] -> w138
            tunnel: w375 -> [w1019]
            tunnel: [w1019] -> w374
            tunnel: w373 -> [w1018]
            tunnel: [w1018] -> w372
            tunnel: w371 -> [w1015]
            tunnel: [w1015] -> w370
            tunnel: w369 -> [w999]
            tunnel: [w999] -> w368
            tunnel: [w999] -> w367
            tunnel: w366 -> [w1017]
            tunnel: [w1017] -> w365
            tunnel: w364 -> [w1016]
            tunnel: [w1016] -> w363
            tunnel: [w999] -> w360
            tunnel: [w999] -> w346
            tunnel: w331 -> [w1014]
            tunnel: [w1014] -> w329
            tunnel: w327 -> [w1013]
            tunnel: [w1013] -> w324
            tunnel: [w1012] -> w308
            tunnel: w307 -> [w1012]
            tunnel: [w1011] -> w305
            tunnel: w304 -> [w1011]
            tunnel: [w1010] -> w303
            tunnel: w302 -> [w1010]
            tunnel: [w1009] -> w289
            tunnel: w288 -> [w1009]
            tunnel: [w1008] -> w260
            tunnel: w259 -> [w1008]
            tunnel: [w1007] -> w242
            tunnel: w241 -> [w1007]
            tunnel: [w1006] -> w238
            tunnel: w237 -> [w1006]
            tunnel: w220 -> [w1005]
            tunnel: [w1005] -> w219
            tunnel: [w1004] -> w217
            tunnel: w216 -> [w1004]
            tunnel: [w1003] -> w215
            tunnel: w213 -> [w1003]
            tunnel: w212 -> [w1002]
            tunnel: [w1002] -> w211
            tunnel: [w1001] -> w177
            tunnel: w176 -> [w1001]
            tunnel: [w1000] -> w175
            tunnel: w174 -> [w1000]
            tunnel: [w999] -> w147
            tunnel: w142 -> [w998]
            tunnel: [w998] -> w141
            tunnel: w140 -> [w997]
            tunnel: [w997] -> w139
            tunnel: w138 -> [w996]
            tunnel: [w996] -> w137
            tunnel: [w1050] -> w345
            tunnel: w374 -> [w1079]
            tunnel: w372 -> [w1078]
            tunnel: w370 -> [w1075]
            tunnel: w368 -> [w1074]
            tunnel: w367 -> [w1073]
            tunnel: w365 -> [w1063]
            tunnel: w363 -> [w1062]
            tunnel: w360 -> [w1064]
            tunnel: [w1060] -> w344
            tunnel: [w1061] -> w343
            tunnel: [w1072] -> w342
            tunnel: [w1071] -> w341
            tunnel: [w1070] -> w340
            tunnel: [w1069] -> w339
            tunnel: w346 -> [w1059]
            tunnel: [w1058] -> w338
            tunnel: [w1057] -> w337
            tunnel: [w1041] -> w336
            tunnel: [w1056] -> w335
            tunnel: w329 -> [w1055]
            tunnel: [w1055] -> w328
            tunnel: [w1054] -> w325
            tunnel: w324 -> [w1054]
            tunnel: w308 -> [w1053]
            tunnel: [w1053] -> w306
            tunnel: w305 -> [w1052]
            tunnel: w303 -> [w1051]
            tunnel: [w1052] -> w301
            tunnel: [w1051] -> w300
            tunnel: w289 -> [w1049]
            tunnel: [w1045] -> w261
            tunnel: w260 -> [w1045]
            tunnel: w242 -> [w1043]
            tunnel: w238 -> [w1042]
            tunnel: [w1036] -> w236
            tunnel: [w1041] -> w235
            tunnel: [w1039] -> w234
            tunnel: [w1037] -> w233
            tunnel: w219 -> [w1040]
            tunnel: [w1040] -> w218
            tunnel: w217 -> [w1039]
            tunnel: w215 -> [w1038]
            tunnel: [w1038] -> w214
            tunnel: w211 -> [w1037]
            tunnel: [w1036] -> w189
            tunnel: [w1035] -> w186
            tunnel: w177 -> [w1034]
            tunnel: w175 -> [w1033]
            tunnel: [w1028] -> w170
            tunnel: [w1029] -> w169
            tunnel: [w1028] -> w168
            tunnel: [w1030] -> w164
            tunnel: [w1029] -> w161
            tunnel: [w1027] -> w158
            tunnel: [w1026] -> w150
            tunnel: w147 -> [w1023]
            tunnel: w141 -> [w1022]
            tunnel: w139 -> [w1021]
            tunnel: w137 -> [w1020]
            tunnel: w345 -> [w1335]
            tunnel: [w1332] -> w319
            tunnel: w344 -> [w1348]
            tunnel: [w1348] -> w318
            tunnel: w343 -> [w1347]
            tunnel: [w1347] -> w317
            tunnel: w342 -> [w1346]
            tunnel: [w1346] -> w316
            tunnel: w341 -> [w1345]
            tunnel: [w1345] -> w315
            tunnel: w340 -> [w1344]
            tunnel: [w1344] -> w314
            tunnel: w339 -> [w1343]
            tunnel: [w1343] -> w313
            tunnel: [w1336] -> w312
            tunnel: w338 -> [w1329]
            tunnel: w337 -> [w1337]
            tunnel: w336 -> [w1336]
            tunnel: w335 -> [w1338]
            tunnel: [w1335] -> w311
            tunnel: w328 -> [w1334]
            tunnel: w325 -> [w1333]
            tunnel: [w1331] -> w310
            tunnel: [w1319] -> w309
            tunnel: w306 -> [w1330]
            tunnel: w301 -> [w1327]
            tunnel: w300 -> [w1326]
            tunnel: [w1328] -> w297
            tunnel: [w1325] -> w294
            tunnel: [w1324] -> w291
            tunnel: [w1320] -> w290
            tunnel: [w1318] -> w262
            tunnel: w261 -> [w1318]
            tunnel: w236 -> [w1317]
            tunnel: w235 -> [w1316]
            tunnel: w234 -> [w1315]
            tunnel: w233 -> [w1313]
            tunnel: [w1311] -> w232
            tunnel: [w1310] -> w231
            tunnel: [w1309] -> w230
            tunnel: [w1308] -> w229
            tunnel: w218 -> [w1312]
            tunnel: w214 -> [w1314]
            tunnel: [w1311] -> w210
            tunnel: [w1310] -> w209
            tunnel: [w1309] -> w208
            tunnel: [w1308] -> w207
            tunnel: [w1307] -> w190
            tunnel: w189 -> [w1307]
            tunnel: [w1306] -> w187
            tunnel: w186 -> [w1306]
            tunnel: w170 -> [w1305]
            tunnel: w169 -> [w1304]
            tunnel: w168 -> [w1303]
            tunnel: [w1303] -> w167
            tunnel: [w1302] -> w165
            tunnel: w164 -> [w1302]
            tunnel: w161 -> [w1301]
            tunnel: [w1301] -> w160
            tunnel: w158 -> [w1300]
            tunnel: [w1300] -> w157
            tunnel: [w1299] -> w151
            tunnel: w150 -> [w1299]
            tunnel: w319 -> [w1384]
            tunnel: [w1391] -> w359
            tunnel: [w1390] -> w358
            tunnel: w318 -> [w1390]
            tunnel: [w1385] -> w355
            tunnel: w317 -> [w1385]
            tunnel: [w1389] -> w353
            tunnel: w316 -> [w1389]
            tunnel: [w1388] -> w351
            tunnel: w315 -> [w1388]
            tunnel: [w1387] -> w349
            tunnel: w314 -> [w1387]
            tunnel: [w1386] -> w347
            tunnel: w313 -> [w1386]
            tunnel: w312 -> [w1373]
            tunnel: w311 -> [w1374]
            tunnel: w310 -> [w1369]
            tunnel: [w1369] -> w322
            tunnel: w309 -> [w1375]
            tunnel: [w1375] -> w320
            tunnel: [w1377] -> w298
            tunnel: w297 -> [w1377]
            tunnel: [w1378] -> w295
            tunnel: w294 -> [w1378]
            tunnel: [w1379] -> w292
            tunnel: w291 -> [w1379]
            tunnel: w290 -> [w1383]
            tunnel: [w1372] -> w263
            tunnel: w262 -> [w1372]
            tunnel: w232 -> [w1368]
            tunnel: w231 -> [w1367]
            tunnel: w230 -> [w1366]
            tunnel: w229 -> [w1365]
            tunnel: w210 -> [w1364]
            tunnel: w209 -> [w1363]
            tunnel: w208 -> [w1362]
            tunnel: w207 -> [w1361]
            tunnel: [w1364] -> w205
            tunnel: [w1363] -> w203
            tunnel: [w1362] -> w201
            tunnel: [w1361] -> w199
            tunnel: w190 -> [w1360]
            tunnel: [w1359] -> w188
            tunnel: w187 -> [w1359]
            tunnel: w167 -> [w1357]
            tunnel: [w1356] -> w166
            tunnel: w165 -> [w1356]
            tunnel: w160 -> [w1355]
            tunnel: w157 -> [w1353]
            tunnel: [w1353] -> w156
            tunnel: [w1352] -> w152
            tunnel: w151 -> [w1352]
            tunnel: w359 -> [w1406]
            tunnel: w358 -> [w1421]
            tunnel: w355 -> [w1415]
            tunnel: w353 -> [w1420]
            tunnel: w351 -> [w1417]
            tunnel: w349 -> [w1419]
            tunnel: w347 -> [w1418]
            tunnel: w322 -> [w1411]
            tunnel: w320 -> [w1410]
            tunnel: w298 -> [w1409]
            tunnel: w295 -> [w1408]
            tunnel: w292 -> [w1407]
            tunnel: [w1400] -> w183
            tunnel: [w1421] -> w275
            tunnel: [w1415] -> w274
            tunnel: [w1420] -> w273
            tunnel: [w1417] -> w272
            tunnel: [w1419] -> w271
            tunnel: [w1418] -> w270
            tunnel: [w1411] -> w269
            tunnel: [w1410] -> w268
            tunnel: [w1409] -> w267
            tunnel: [w1408] -> w266
            tunnel: [w1407] -> w265
            tunnel: [w1405] -> w264
            tunnel: w263 -> [w1405]
            tunnel: [w1404] -> w206
            tunnel: w205 -> [w1404]
            tunnel: [w1403] -> w204
            tunnel: w203 -> [w1403]
            tunnel: [w1402] -> w202
            tunnel: w201 -> [w1402]
            tunnel: [w1401] -> w200
            tunnel: w199 -> [w1401]
            tunnel: w188 -> [w1399]
            tunnel: [w1398] -> w173
            tunnel: [w1397] -> w172
            tunnel: w166 -> [w1396]
            tunnel: [w1395] -> w163
            tunnel: [w1394] -> w162
            tunnel: w156 -> [w1393]
            tunnel: [w1393] -> w155
            tunnel: [w1392] -> w153
            tunnel: w152 -> [w1392]
            tunnel: w275 -> [w1469]
            tunnel: w274 -> [w1468]
            tunnel: w273 -> [w1467]
            tunnel: w272 -> [w1466]
            tunnel: w271 -> [w1465]
            tunnel: w270 -> [w1464]
            tunnel: w269 -> [w1463]
            tunnel: w268 -> [w1462]
            tunnel: w267 -> [w1461]
            tunnel: w266 -> [w1460]
            tunnel: w265 -> [w1459]
            tunnel: w264 -> [w1454]
            tunnel: [w1469] -> w257
            tunnel: [w1468] -> w256
            tunnel: [w1467] -> w255
            tunnel: [w1466] -> w254
            tunnel: [w1465] -> w253
            tunnel: [w1464] -> w252
            tunnel: [w1463] -> w251
            tunnel: [w1462] -> w250
            tunnel: [w1461] -> w249
            tunnel: [w1460] -> w248
            tunnel: [w1459] -> w247
            tunnel: [w1454] -> w246
            tunnel: [w1453] -> w245
            tunnel: w206 -> [w1452]
            tunnel: w204 -> [w1451]
            tunnel: w202 -> [w1450]
            tunnel: w200 -> [w1449]
            tunnel: [w1452] -> w198
            tunnel: [w1451] -> w196
            tunnel: [w1450] -> w194
            tunnel: [w1449] -> w192
            tunnel: w173 -> [w1448]
            tunnel: w172 -> [w1447]
            tunnel: [w1442] -> w171
            tunnel: w163 -> [w1441]
            tunnel: w162 -> [w1440]
            tunnel: w155 -> [w1437]
            tunnel: [w1437] -> w154
            tunnel: w153 -> [w1436]
            tunnel: [w1436] -> w148
            tunnel: [w1482] -> w293
            tunnel: [w1483] -> w296
            tunnel: [w1484] -> w299
            tunnel: [w1485] -> w321
            tunnel: [w1486] -> w323
            tunnel: [w1487] -> w348
            tunnel: [w1488] -> w350
            tunnel: [w1489] -> w352
            tunnel: [w1490] -> w354
            tunnel: [w1491] -> w356
            tunnel: [w1492] -> w357
            tunnel: w257 -> [w1492]
            tunnel: w256 -> [w1491]
            tunnel: w255 -> [w1490]
            tunnel: w254 -> [w1489]
            tunnel: w253 -> [w1488]
            tunnel: w252 -> [w1487]
            tunnel: w251 -> [w1486]
            tunnel: w250 -> [w1485]
            tunnel: w249 -> [w1484]
            tunnel: w248 -> [w1483]
            tunnel: w247 -> [w1482]
            tunnel: w246 -> [w1478]
            tunnel: w245 -> [w1477]
            tunnel: [w1476] -> w197
            tunnel: w198 -> [w1476]
            tunnel: [w1475] -> w195
            tunnel: w196 -> [w1475]
            tunnel: [w1474] -> w193
            tunnel: w194 -> [w1474]
            tunnel: [w1473] -> w191
            tunnel: w192 -> [w1473]
            tunnel: [w1472] -> w185
            tunnel: w171 -> [w1472]
            tunnel: [w1471] -> w159
            tunnel: w154 -> [w1471]
            tunnel: [w1470] -> w149
            tunnel: w148 -> [w1470]
            frame #0 {
              n17 = Tick Count (ms)() -> (millisecond timer value=w389:u32)
            }
            frame #1 {
              n18 = while {
                tunnel: "Keithley delay (ms)" -> [w435]
                tunnel: w405 -> [w434]
                tunnel: w404 -> [w433]
                tunnel: [w430] -> w402
                tunnel: [w429] -> w401
                stop <- w431 stop-if-true
                n19 = event shown="[1] \"Set Output Current\": Value Change" {
                  selector: _ -> [_ _]
                  dyn-events: _ -> [_ _]
                  timeout: 1 -> [_ _]
                  tunnel: w435 -> [_ w441]
                  tunnel: w434 -> [w437 w440]
                  tunnel: w433 -> [w436 w439]
                  tunnel: [TRUE _] -> w431
                  tunnel: [w437 w440] -> w430
                  tunnel: [w436 w439] -> w429
                  event Timeout {
                    n20 = event-data() -> ()  [unwired: 1 in, 2 out]
                  }
                  event "Set Output Current": Value Change {
                    n21 = event-data() -> ()  [unwired: 1 in, 5 out]
                    n22 = for {
                      N: 2 -> [_]
                      tunnel: w441 -> [w445]
                      tunnel: w440 -> [w444]
                      tunnel: w439 -> [w443]
                      i -> [w448]
                      n23 = flat-sequence {
                        tunnel: [w455] -> w450
                        tunnel: w448 -> [w454]
                        tunnel: [w453] -> w447
                        tunnel: w444 -> [w452]
                        tunnel: w443 -> [w451]
                        tunnel: w450 -> [w476]
                        tunnel: [w476] -> w449
                        tunnel: w447 -> [w475]
                        tunnel: [w475] -> w446
                        tunnel: w445 -> [w474]
                        tunnel: w449 -> [w481]
                        tunnel: w448 -> [w480]
                        tunnel: w446 -> [w479]
                        tunnel: [w478] -> _
                        tunnel: [w477] -> _
                        frame #0 {
                          n24 = case shown="0, Default" w454 {
                            tunnel: [w468 w470] -> w455
                            tunnel: [w467 w469] -> w453
                            tunnel: w452 -> [w466 w472]
                            tunnel: w451 -> [w465 w473]
                            frame 0, Default {
                              n25 = Multiply(x="output current setpoint (A)", y=0.001) -> (x*y=w457:dbl)
                              n26 = Number To Exponential String(number=w457, 1:FALSE ("use system decimal point (T)")) -> (E-format string=w463:string)  [unwired: 2 in]
                              n27 = Concatenate Strings("SOUR:CURR " ("string"), w463) -> (w461:string)
                              n28 = Concatenate Strings(w461, "\n" ("string")) -> (w460:string)
                              "command to Keithley" <- w460
                              n29 = VISA Write(VISA resource name=w466, write buffer=w460, error in (no error)=w465) -> (VISA resource name out=w468:refnum<visa-resource-name>, error out=w467:errorcluster)  [unwired: 1 out]
                            }
                            frame 1 {
                              n30 = VISA Write(VISA resource name=w472, write buffer="SOUR:CURR?\n" ("string"), error in (no error)=w473) -> (VISA resource name out=w470:refnum<visa-resource-name>, error out=w469:errorcluster)  [unwired: 1 out]
                            }
                          }
                        }
                        frame #1 {
                          n31 = Wait (ms)(milliseconds to wait=w474) -> ()  [unwired: 1 out]
                        }
                        frame #2 {
                          n32 = case shown="0, Default" w480 {
                            tunnel: w481 -> [w483 w487]
                            tunnel: w479 -> [w482 w486]
                            tunnel: [w483 w485] -> w478
                            tunnel: [w482 w484] -> w477
                            frame 0, Default {
                            }
                            frame 1 {
                              n33 = property class="Instr"(reference=w487, error in=w486) -> (reference out=w489:refnum<visa-resource-name>, error out=w488:errorcluster, "Bytes at Port"=w491:u32)
                              "Bytes at Port" <- w491
                              n34 = VISA Read(VISA resource name=w489, byte count=w491, error in (no error)=w488) -> (VISA resource name out=w485:refnum<visa-resource-name>, read buffer=→"actual value":string, error out=w484:errorcluster)  [unwired: 1 out]
                            }
                          }
                        }
                      }
                    }
                  }
                }
              }
              n35 = while {
                tunnel: w426 -> [w496]
                tunnel: [w495] -> w425
                tunnel: [w494] -> w424
                tunnel: w412 -> [w492]
                stop <- w497 stop-if-true
                n36 = event shown="[7] \"Set PID\": Value Change" {
                  selector: _ -> [_ _ _ _ _ _ _ _ _ _ _ _]
                  dyn-events: _ -> [_ _ _ _ _ _ _ _ _ _ _ _]
                  timeout: 1 -> [_ _ _ _ _ _ _ _ _ _ _ _]
                  tunnel: [TRUE ("Set Gauge to Zero") w505 w554 w575 w601 w636 w692 w743 w822 w893 "Set Gauge to Zero" _] -> w497
                  tunnel: w496 -> [w501 w504 w551 w573 w597 w635 w688 w741 w820 w891 w968 w990]
                  tunnel: [w500 w503 w550 w572 w599 w633 w690 w740 w819 w890 w967 w989] -> w495
                  tunnel: [w499 w502 w549 w571 w598 w634 w689 w739 w818 w889 w966 w988] -> w494
                  tunnel: w492 -> [_ _ _ _ _ _ _ _ _ _ w964 _]
                  event Timeout {
                    n37 = event-data() -> ()  [unwired: 1 in, 1 out]
                    n38 = Unbundle(w501) -> ("VISA resource name out"=w500:refnum<visa-resource-name>, "error out"=w499:errorcluster)  [unwired: 2 out]
                  }
                  event "Setpoint\n START": Value Change {
                    n39 = event-data() -> ()  [unwired: 1 in, 1 out]
                    n40 = stacked-sequence {
                      tunnel: w504 -> [_ w511 _]
                      tunnel: [_ w510 _] -> w502
                      tunnel: [_ w509 _] -> w503
                      frame #0 {
                        n41 = property on="Setpoint\n START" class="Bool"("Blinking"=TRUE) -> ()  [unwired: 2 in, 2 out]
                        n42 = property on="ON" class="Bool (strict)"("Blinking"=FALSE) -> ()  [unwired: 2 in, 2 out]
                      }
                      frame #1 {
                        n43 = for {
                          N: 2 -> [_]
                          tunnel: w511 -> [w515]
                          tunnel: [w514] -> w510
                          tunnel: [w513] -> w509
                          i -> [w517]
                          n44 = flat-sequence {
                            tunnel: [w520] -> w516
                            tunnel: w517 -> [w519]
                            tunnel: [w538] -> w518
                            tunnel: w516 -> [w537]
                            tunnel: w515 -> [w539]
                            tunnel: [w536] -> w514
                            tunnel: [w535] -> w513
                            tunnel: w518 -> [w545]
                            tunnel: w517 -> [w544]
                            frame #0 {
                              n45 = case shown="0, Default" w519 {
                                tunnel: [w529 w531] -> w520
                                frame 0, Default {
                                n46 = Multiply(x=10.0, y="SP 1 input (°C)") -> (x*y=w526:dbl)
                                n47 = local read "RAM"() -> (w524:bool)
                                n48 = Number To Hexadecimal String(1:i16 5 ("width (-)"), 2:w526) -> (0:w528:string)
                                n49 = Select(t="*P012", s=w524, f="*P012") -> (s? t:f=w521:string)
                                n50 = Concatenate Strings(w521, w528) -> (w529:string)
                                }
                                frame 1 {
                                n51 = local read "RAM"() -> (w534:bool)
                                n52 = Select(t="*G01", s=w534, f="*R01") -> (s? t:f=w531:string)
                                }
                              }
                            }
                            frame #1 {
                              n53 = Unbundle(w539) -> ("VISA resource name out"=w540:refnum<visa-resource-name>, "error out"=w542:errorcluster, "Delay (ms)"=w541:u32, "Write/\nRead"=w543:bool)
                              n54 = call "I3252_Comm_Interface.vi"("VISA resource name in"=w540, "error in"=w542, "Delay (ms)"=w541, "Write"=w543, "String to Write"=w537, "Read"=w543) -> ("VISA resource name out"=w535:refnum<visa-resource-name>, "error out"=w536:errorcluster, "Read String"=w538:string)  [unwired: 2 in]
                            }
                            frame #2 {
                              n55 = case shown="0, Default" w544 {
                                tunnel: w545 -> [_ w547]
                                frame 0, Default {
                                }
                                frame 1 {
                                n56 = call "I3252_Edit_Setpoint.vi"("Read String"=w547) -> ("Setpoint is"=→"SP 1 is (°C)":dbl)
                                }
                              }
                            }
                          }
                        }
                      }
                      frame #2 {
                        n57 = property on="Setpoint\n START" class="Bool"("Blinking"=FALSE) -> ()  [unwired: 2 in, 2 out]
                      }
                    }
                    n58 = Not(x="Setpoint\n START") -> (.not. x?=w505:bool)
                  }
                  event "Standby": Value Change {
                    n59 = event-data() -> ()  [unwired: 1 in, 1 out]
                    n60 = flat-sequence {
                      tunnel: [w562] -> w552
                      tunnel: w552 -> [w566]
                      tunnel: w551 -> [w565]
                      tunnel: [w564] -> w549
                      tunnel: [w563] -> w550
                      frame #0 {
                        n61 = local read "Standby"() -> (w555:bool)
                        n62 = Select(t=TRUE, s=w555, f=FALSE) -> (s? t:f=w558:bool)
                        n63 = property on="Standby" class="Bool (strict)"("Blinking"=w558) -> ()  [unwired: 2 in, 2 out]
                      }
                      frame #1 {
                        n64 = local read "Standby"() -> (w560:bool)
                        n65 = Select(t="*D03", s=w560, f="*E03") -> (s? t:f=w562:string)
                      }
                      frame #2 {
                        n66 = Unbundle(w565) -> ("VISA resource name out"=w567:refnum<visa-resource-name>, "error out"=w569:errorcluster, "Delay (ms)"=w568:u32, "Write/\nRead"=w570:bool)
                        n67 = call "I3252_Comm_Interface.vi"("VISA resource name in"=w567, "error in"=w569, "Delay (ms)"=w568, "Write"=w570, "String to Write"=w566, "Read"=w570) -> ("VISA resource name out"=w563:refnum<visa-resource-name>, "error out"=w564:errorcluster)  [unwired: 2 in, 1 out]
                      }
                    }
                    n68 = Not(x="Standby") -> (.not. x?=w554:bool)
                  }
                  event "Set Command": Value Change {
                    n69 = event-data() -> ()  [unwired: 1 in, 1 out]
                    n70 = stacked-sequence {
                      tunnel: w573 -> [_ w580 _]
                      tunnel: [_ w579 _] -> w572
                      tunnel: [_ w578 _] -> w571
                      frame #0 {
                        n71 = property on="Set Command" class="Bool"("Blinking"=TRUE) -> ()  [unwired: 2 in, 2 out]
                        n72 = property on="ON" class="Bool (strict)"("Blinking"=FALSE) -> ()  [unwired: 2 in, 2 out]
                      }
                      frame #1 {
                        n73 = flat-sequence {
                          tunnel: [w585] -> w582
                          tunnel: [w588] -> w581
                          tunnel: w582 -> [w589]
                          tunnel: w580 -> [w590]
                          tunnel: [w587] -> w579
                          tunnel: [w586] -> _
                          tunnel: [w586] -> w578
                          tunnel: w581 -> [w595]
                          frame #0 {
                            n74 = Concatenate Strings("*", "Command input") -> (w585:string)
                          }
                          frame #1 {
                            n75 = Unbundle(w590) -> ("VISA resource name out"=w594:refnum<visa-resource-name>, "error out"=w592:errorcluster, "Delay (ms)"=w593:u32, "Write/\nRead"=w591:bool)
                            n76 = call "I3252_Comm_Interface.vi"("VISA resource name in"=w594, "error in"=w592, "Delay (ms)"=w593, "Write"=w591, "String to Write"=w589, "Read"=w591) -> ("VISA resource name out"=w587:refnum<visa-resource-name>, "error out"=w586:errorcluster, "Read String"=w588:string)  [unwired: 2 in]
                          }
                          frame #2 {
                            "Command output" <- w595
                          }
                        }
                      }
                      frame #2 {
                        n77 = property on="Set Command" class="Bool"("Blinking"=FALSE) -> ()  [unwired: 2 in, 2 out]
                      }
                    }
                    n78 = Not(x="Set Command") -> (.not. x?=w575:bool)
                  }
                  event "Reset\nSTOPP": Value Change {
                    n79 = event-data() -> ()  [unwired: 1 in, 1 out]
                    n80 = stacked-sequence {
                      tunnel: [_ w608 _] -> w598
                      tunnel: [_ w607 _] -> w599
                      tunnel: w597 -> [_ w605 _]
                      frame #0 {
                        n81 = property on="Reset\nSTOPP" class="Bool"("Blinking"=TRUE) -> ()  [unwired: 2 in, 2 out]
                        n82 = property on="ON" class="Bool (strict)"("Blinking"=FALSE) -> ()  [unwired: 2 in, 2 out]
                      }
                      frame #1 {
                        n83 = for {
                          N: 2 -> [_]
                          tunnel: [w614] -> w608
                          tunnel: [w613] -> w607
                          tunnel: w605 -> [w612]
                          i -> [w610]
                          n84 = flat-sequence {
                            tunnel: w610 -> [w616]
                            tunnel: [w615] -> w611
                            tunnel: [w621] -> w614
                            tunnel: [w622] -> w613
                            tunnel: w612 -> [w623]
                            tunnel: w611 -> [w620]
                            tunnel: [w619] -> w609
                            tunnel: w610 -> [w629]
                            tunnel: w609 -> [w628]
                            frame #0 {
                              n85 = case shown="0, Default" w616 {
                                tunnel: ["*Z02" "*G01"] -> w615
                                frame 0, Default {
                                }
                                frame 1 {
                                }
                              }
                            }
                            frame #1 {
                              n86 = Unbundle(w623) -> ("VISA resource name out"=w624:refnum<visa-resource-name>, "error out"=w626:errorcluster, "Delay (ms)"=w625:u32, "Write/\nRead"=w627:bool)
                              n87 = call "I3252_Comm_Interface.vi"("VISA resource name in"=w624, "error in"=w626, "Delay (ms)"=w625, "Write"=w627, "String to Write"=w620, "Read"=w627) -> ("VISA resource name out"=w622:refnum<visa-resource-name>, "error out"=w621:errorcluster, "Read String"=w619:string)  [unwired: 2 in]
                            }
                            frame #2 {
                              n88 = case shown="0, Default" w629 {
                                tunnel: w628 -> [_ w631]
                                frame 0, Default {
                                }
                                frame 1 {
                                n89 = call "I3252_Edit_Setpoint.vi"("Read String"=w631) -> ("Setpoint is"=w630:dbl)
                                n90 = local write "SP 1 is (°C)"(w630) -> ()
                                }
                              }
                            }
                          }
                        }
                        n91 = Wait (ms)(milliseconds to wait=u32 4000) -> ()  [unwired: 1 out]
                      }
                      frame #2 {
                        n92 = property on="Reset\nSTOPP" class="Bool"("Blinking"=FALSE) -> ()  [unwired: 2 in, 2 out]
                      }
                    }
                    n93 = Not(x="Reset\nSTOPP") -> (.not. x?=w601:bool)
                  }
                  event "Auto Tune": Value Change {
                    n94 = event-data() -> ()  [unwired: 1 in, 1 out]
                    n95 = stacked-sequence {
                      tunnel: w635 -> [_ w642 w687]
                      tunnel: [_ w641 _] -> w634
                      tunnel: [_ w640 _] -> w633
                      frame #0 {
                        n96 = property on="Auto Tune" class="Bool"("Blinking"=TRUE) -> ()  [unwired: 2 in, 2 out]
                        n97 = property on="ON" class="Bool (strict)"("Blinking"=FALSE) -> ()  [unwired: 2 in, 2 out]
                      }
                      frame #1 {
                        n98 = for {
                          N: 4 -> [_]
                          tunnel: [w647] -> w640
                          tunnel: [w646] -> w641
                          tunnel: w642 -> [w645]
                          i -> [w650]
                          n99 = flat-sequence {
                            tunnel: w650 -> [w652]
                            tunnel: [w651] -> w648
                            tunnel: w648 -> [w667]
                            tunnel: [w666] -> w649
                            tunnel: [w669] -> w647
                            tunnel: [w668] -> w646
                            tunnel: w645 -> [w665]
                            tunnel: w650 -> [w675]
                            tunnel: w649 -> [w674]
                            frame #0 {
                              n100 = case shown="0, Default" w652 {
                                tunnel: ["*V01" w655 "*W0C35" "*Z02"] -> w651
                                frame 0, Default {
                                }
                                frame 1 {
                                n101 = local read "(°C)"() -> (w654:dbl)
                                n102 = Add(x=20.0, y=w654) -> (x+y=w661:dbl)
                                n103 = Multiply(x=10.0, y=w661) -> (x*y=w658:dbl)
                                n104 = Number To Hexadecimal String(1:i16 5 ("width (-)"), 2:w658) -> (0:w657:string)
                                n105 = Concatenate Strings("*W012", w657) -> (w655:string)
                                }
                                frame 2 {
                                # "35 hex = \n00110101 bin"
                                }
                                frame 3 {
                                }
                              }
                            }
                            frame #1 {
                              n106 = Unbundle(w665) -> ("VISA resource name out"=w673:refnum<visa-resource-name>, "error out"=w671:errorcluster, "Delay (ms)"=w672:u32, "Write/\nRead"=w670:bool)
                              n107 = call "I3252_Comm_Interface.vi"("VISA resource name in"=w673, "error in"=w671, "Delay (ms)"=w672, "Write"=w670, "String to Write"=w667, "Read"=w670) -> ("VISA resource name out"=w669:refnum<visa-resource-name>, "error out"=w668:errorcluster, "Read String"=w666:string)  [unwired: 2 in]
                            }
                            frame #2 {
                              n108 = case shown="0, Default" w675 {
                                tunnel: w674 -> [w677]
                                frame 0, Default {
                                n109 = call <vilib>:"Space Constant.vi"() -> ("String"=w680:string)
                                n110 = Search/Split String(string=w677, search string/char (-)=w680) -> (match + rest of string=w679:string)  [unwired: 1 in, 2 out]
                                n111 = Fract/Exp String To Number(use system decimal point (T)=FALSE, string=w679) -> (number=w676:dbl)  [unwired: 2 in, 1 out]
                                n112 = local write "(°C)"(w676) -> ()
                                }
                              }
                            }
                          }
                        }
                        n113 = Wait (ms)(milliseconds to wait=u32 45000) -> ()  [unwired: 1 out]
                      }
                      frame #2 {
                        n114 = Unbundle(w687) -> ("VISA resource name out"=w686:refnum<visa-resource-name>, "error out"=w684:errorcluster, "Delay (ms)"=w685:u32, "Write/\nRead"=w683:bool)
                        n115 = property on="Auto Tune" class="Bool"("Blinking"=FALSE) -> ()  [unwired: 2 in, 2 out]
                        n116 = call "I3252_Comm_Interface.vi"("VISA resource name in"=w686, "error in"=w684, "Delay (ms)"=w685, "Write"=w683, "String to Write"="*W01200000", "Read"=w683) -> ()  [unwired: 2 in, 3 out]
                      }
                    }
                    n117 = Not(x="Auto Tune") -> (.not. x?=w636:bool)
                  }
                  event "Write LOW/HI": Value Change {
                    n118 = event-data() -> ()  [unwired: 1 in, 1 out]
                    n119 = stacked-sequence {
                      tunnel: [_ w697 _] -> w690
                      tunnel: [_ w696 _] -> w689
                      tunnel: w688 -> [_ w695 _]
                      frame #0 {
                        n120 = property on="Write LOW/HI" class="Bool"("Blinking"=TRUE) -> ()  [unwired: 2 in, 2 out]
                        n121 = property on="ON" class="Bool (strict)"("Blinking"=FALSE) -> ()  [unwired: 2 in, 2 out]
                      }
                      frame #1 {
                        n122 = for {
                          N: 4 -> [_]
                          tunnel: [w701] -> w697
                          tunnel: [w700] -> w696
                          tunnel: w695 -> [w699]
                          i -> [w703]
                          n123 = flat-sequence {
                            tunnel: w703 -> [w705]
                            tunnel: [w706] -> w702
                            tunnel: w702 -> [w720]
                            tunnel: [w721] -> w704
                            tunnel: [w723] -> w701
                            tunnel: [w722] -> w700
                            tunnel: w699 -> [w719]
                            tunnel: w704 -> [w729]
                            tunnel: w703 -> [w728]
                            frame #0 {
                              n124 = case shown="1" w705 {
                                tunnel: [w708 w714 "*R27" "*R28"] -> w706
                                frame 0, Default {
                                n125 = Number To Hexadecimal String(1:i16 2 ("width (-)"), 2:"% LOW Sollwert") -> (0:w709:string)
                                n126 = Concatenate Strings("*W27", w709) -> (w708:string)
                                }
                                frame 1 {
                                n127 = Number To Hexadecimal String(1:i16 2 ("width (-)"), 2:"% High Sollwert") -> (0:w715:string)
                                n128 = Concatenate Strings("*W28", w715) -> (w714:string)
                                }
                                frame 2 {
                                }
                                frame 3 {
                                }
                              }
                            }
                            frame #1 {
                              n129 = Unbundle(w719) -> ("VISA resource name out"=w727:refnum<visa-resource-name>, "error out"=w725:errorcluster, "Delay (ms)"=w726:u32, "Write/\nRead"=w724:bool)
                              n130 = call "I3252_Comm_Interface.vi"("VISA resource name in"=w727, "error in"=w725, "Delay (ms)"=w726, "Write"=w724, "String to Write"=w720, "Read"=w724) -> ("VISA resource name out"=w723:refnum<visa-resource-name>, "error out"=w722:errorcluster, "Read String"=w721:string)  [unwired: 2 in]
                            }
                            frame #2 {
                              n131 = case shown="0, Default" w728 {
                                tunnel: w729 -> [_ w733 w737]
                                frame 0, Default {
                                }
                                frame 2 {
                                n132 = String Subset(string=w733, offset (0)=3) -> (substring=w731:string)  [unwired: 1 in]
                                n133 = Hexadecimal String To Number(string=w731) -> (number=→"% LOW Istwert":u32)  [unwired: 2 in, 1 out]
                                }
                                frame 3 {
                                n134 = String Subset(string=w737, offset (0)=3) -> (substring=w735:string)  [unwired: 1 in]
                                n135 = Hexadecimal String To Number(string=w735) -> (number=→"% HIGH Istwert":u32)  [unwired: 2 in, 1 out]
                                }
                              }
                            }
                          }
                        }
                      }
                      frame #2 {
                        n136 = property on="Write LOW/HI" class="Bool"("Blinking"=FALSE) -> ()  [unwired: 2 in, 2 out]
                      }
                    }
                    n137 = Not(x="Write LOW/HI") -> (.not. x?=w692:bool)
                  }
                  event "Set PID": Value Change {
                    n138 = event-data() -> ()  [unwired: 1 in, 1 out]
                    n139 = stacked-sequence {
                      tunnel: w741 -> [_ w748 _]
                      tunnel: [_ w747 _] -> w740
                      tunnel: [_ w746 _] -> w739
                      frame #0 {
                        n140 = property on="Set PID" class="Bool"("Blinking"=TRUE) -> ()  [unwired: 2 in, 2 out]
                        n141 = property on="ON" class="Bool (strict)"("Blinking"=FALSE) -> ()  [unwired: 2 in, 2 out]
                      }
                      frame #1 {
                        n142 = for {
                          N: 6 -> [_]
                          tunnel: w748 -> [w752]
                          tunnel: [w751] -> w747
                          tunnel: [w750] -> w746
                          i -> [w754]
                          n143 = flat-sequence {
                            tunnel: w754 -> [w756]
                            tunnel: [w757] -> w753
                            tunnel: w753 -> [w798]
                            tunnel: [w794] -> w755
                            tunnel: w752 -> [w797]
                            tunnel: [w796] -> w750
                            tunnel: [w795] -> w751
                            tunnel: w755 -> [w804]
                            tunnel: w754 -> [w803]
                            frame #0 {
                              n144 = case shown="3" w756 {
                                tunnel: [w764 w772 w780 w782 w786 w790] -> w757
                                frame 0, Default {
                                n145 = local read "RAM"() -> (w758:bool)
                                n146 = Number To Hexadecimal String(1:i16 4 ("width (-)"), 2:"P (PB1) Sollwert") -> (0:w765:string)
                                n147 = Select(t="*P17", s=w758, f="*W17") -> (s? t:f=w759:string)
                                n148 = Concatenate Strings(w759, w765) -> (w764:string)
                                }
                                frame 1 {
                                n149 = local read "RAM"() -> (w766:bool)
                                n150 = Number To Hexadecimal String(1:i16 4 ("width (-)"), 2:"I ( Reset1) Sollwert") -> (0:w773:string)
                                n151 = Select(t="*P18", s=w766, f="*W18") -> (s? t:f=w768:string)
                                n152 = Concatenate Strings(w768, w773) -> (w772:string)
                                }
                                frame 2 {
                                n153 = local read "RAM"() -> (w775:bool)
                                n154 = Number To Hexadecimal String(1:i16 4 ("width (-)"), 2:"D (Rate) Sollwert") -> (0:w781:string)
                                n155 = Select(t="*P19", s=w775, f="*W19") -> (s? t:f=w776:string)
                                n156 = Concatenate Strings(w776, w781) -> (w780:string)
                                }
                                frame 3 {
                                n157 = local read "RAM"() -> (w785:bool)
                                n158 = Select(t="*G17", s=w785, f="*R17") -> (s? t:f=w782:string)
                                }
                                frame 4 {
                                n159 = local read "RAM"() -> (w789:bool)
                                n160 = Select(t="*G18", s=w789, f="*R18") -> (s? t:f=w786:string)
                                }
                                frame 5 {
                                n161 = local read "RAM"() -> (w793:bool)
                                n162 = Select(t="*G19", s=w793, f="*R19") -> (s? t:f=w790:string)
                                }
                              }
                            }
                            frame #1 {
                              n163 = Unbundle(w797) -> ("VISA resource name out"=w802:refnum<visa-resource-name>, "error out"=w800:errorcluster, "Delay (ms)"=w801:u32, "Write/\nRead"=w799:bool)
                              n164 = call "I3252_Comm_Interface.vi"("VISA resource name in"=w802, "error in"=w800, "Delay (ms)"=w801, "Write"=w799, "String to Write"=w798, "Read"=w799) -> ("VISA resource name out"=w795:refnum<visa-resource-name>, "error out"=w796:errorcluster, "Read String"=w794:string)  [unwired: 2 in]
                            }
                            frame #2 {
                              n165 = case shown="3" w803 {
                                tunnel: w804 -> [_ w808 w812 w816]
                                frame 0, Default {
                                }
                                frame 3 {
                                n166 = String Subset(string=w808, offset (0)=3) -> (substring=w806:string)  [unwired: 1 in]
                                n167 = Hexadecimal String To Number(string=w806) -> (number=→"P (PB1) Istwert":u32)  [unwired: 2 in, 1 out]
                                }
                                frame 4 {
                                n168 = String Subset(string=w812, offset (0)=3) -> (substring=w810:string)  [unwired: 1 in]
                                n169 = Hexadecimal String To Number(string=w810) -> (number=→"I ( Reset1) Istwert":u32)  [unwired: 2 in, 1 out]
                                }
                                frame 5 {
                                n170 = String Subset(string=w816, offset (0)=3) -> (substring=w814:string)  [unwired: 1 in]
                                n171 = Hexadecimal String To Number(string=w814) -> (number=→"D (Rate) IstWert":u32)  [unwired: 2 in, 1 out]
                                }
                              }
                            }
                          }
                        }
                      }
                      frame #2 {
                        n172 = property on="Set PID" class="Bool"("Blinking"=FALSE) -> ()  [unwired: 2 in, 2 out]
                      }
                    }
                    n173 = Not(x="Set PID") -> (.not. x?=w743:bool)
                  }
                  event "Get Values": Value Change {
                    n174 = event-data() -> ()  [unwired: 1 in, 1 out]
                    n175 = stacked-sequence {
                      tunnel: w820 -> [_ w827 _]
                      tunnel: [_ w826 _] -> w819
                      tunnel: [_ w825 _] -> w818
                      frame #0 {
                        n176 = property on="Get Values" class="Bool"("Blinking"=TRUE) -> ()  [unwired: 2 in, 2 out]
                        n177 = property on="ON" class="Bool (strict)"("Blinking"=FALSE) -> ()  [unwired: 2 in, 2 out]
                      }
                      frame #1 {
                        n178 = for {
                          N: 6 -> [_]
                          tunnel: w827 -> [w831]
                          tunnel: [w830] -> w826
                          tunnel: [w829] -> w825
                          i -> [w833]
                          n179 = flat-sequence {
                            tunnel: w833 -> [w835]
                            tunnel: [w836] -> w832
                            tunnel: w832 -> [w858]
                            tunnel: [w859] -> w834
                            tunnel: w831 -> [w857]
                            tunnel: [w856] -> w829
                            tunnel: [w855] -> w830
                            tunnel: w834 -> [w865]
                            tunnel: w833 -> [w864]
                            frame #0 {
                              n180 = case shown="0, Default" w835 {
                                tunnel: [w839 w843 w847 "*R27" "*R28" w853] -> w836
                                frame 0, Default {
                                n181 = local read "RAM"() -> (w840:bool)
                                n182 = Select(t="*G17", s=w840, f="*R17") -> (s? t:f=w839:string)
                                }
                                frame 1 {
                                n183 = local read "RAM"() -> (w844:bool)
                                n184 = Select(t="*G18", s=w844, f="*R18") -> (s? t:f=w843:string)
                                }
                                frame 2 {
                                n185 = local read "RAM"() -> (w848:bool)
                                n186 = Select(t="*G19", s=w848, f="*R19") -> (s? t:f=w847:string)
                                }
                                frame 3 {
                                }
                                frame 4 {
                                }
                                frame 5 {
                                n187 = local read "RAM"() -> (w854:bool)
                                n188 = Select(t="*G01", s=w854, f="*R01") -> (s? t:f=w853:string)
                                }
                              }
                            }
                            frame #1 {
                              n189 = Unbundle(w857) -> ("VISA resource name out"=w863:refnum<visa-resource-name>, "error out"=w861:errorcluster, "Delay (ms)"=w862:u32, "Write/\nRead"=w860:bool)
                              n190 = call "I3252_Comm_Interface.vi"("VISA resource name in"=w863, "error in"=w861, "Delay (ms)"=w862, "Write"=w860, "String to Write"=w858, "Read"=w860) -> ("VISA resource name out"=w855:refnum<visa-resource-name>, "error out"=w856:errorcluster, "Read String"=w859:string)  [unwired: 2 in]
                            }
                            frame #2 {
                              n191 = case shown="0, Default" w864 {
                                tunnel: w865 -> [w867 w871 w875 w879 w883 w887]
                                frame 0, Default {
                                n192 = String Subset(string=w867, offset (0)=3) -> (substring=w868:string)  [unwired: 1 in]
                                n193 = Hexadecimal String To Number(string=w868) -> (number=w866:u32)  [unwired: 2 in, 1 out]
                                n194 = local write "P (PB1) Sollwert"(w866) -> ()
                                n195 = local write "P (PB1) Istwert"(w866) -> ()
                                }
                                frame 1 {
                                n196 = String Subset(string=w871, offset (0)=3) -> (substring=w872:string)  [unwired: 1 in]
                                n197 = Hexadecimal String To Number(string=w872) -> (number=w870:u32)  [unwired: 2 in, 1 out]
                                n198 = local write "I ( Reset1) Sollwert"(w870) -> ()
                                n199 = local write "I ( Reset1) Istwert"(w870) -> ()
                                }
                                frame 2 {
                                n200 = String Subset(string=w875, offset (0)=3) -> (substring=w876:string)  [unwired: 1 in]
                                n201 = Hexadecimal String To Number(string=w876) -> (number=w874:u32)  [unwired: 2 in, 1 out]
                                n202 = local write "D (Rate) Sollwert"(w874) -> ()
                                n203 = local write "D (Rate) IstWert"(w874) -> ()
                                }
                                frame 3 {
                                n204 = String Subset(string=w879, offset (0)=3) -> (substring=w880:string)  [unwired: 1 in]
                                n205 = Hexadecimal String To Number(string=w880) -> (number=w878:u32)  [unwired: 2 in, 1 out]
                                n206 = local write "% LOW Istwert"(w878) -> ()
                                n207 = local write "% LOW Sollwert"(w878) -> ()
                                }
                                frame 4 {
                                n208 = String Subset(string=w883, offset (0)=3) -> (substring=w884:string)  [unwired: 1 in]
                                n209 = Hexadecimal String To Number(string=w884) -> (number=w882:u32)  [unwired: 2 in, 1 out]
                                n210 = local write "% High Sollwert"(w882) -> ()
                                n211 = local write "% HIGH Istwert"(w882) -> ()
                                }
                                frame 5 {
                                n212 = call "I3252_Edit_Setpoint.vi"("Read String"=w887) -> ("Setpoint is"=w886:dbl)
                                n213 = local write "SP 1 is (°C)"(w886) -> ()
                                }
                              }
                            }
                          }
                        }
                      }
                      frame #2 {
                        n214 = property on="Get Values" class="Bool"("Blinking"=FALSE) -> ()  [unwired: 2 in, 2 out]
                      }
                    }
                    n215 = Not(x="Get Values") -> (.not. x?=w822:bool)
                  }
                  event "RAM": Value Change {
                    n216 = event-data() -> ()  [unwired: 1 in, 1 out]
                    n217 = stacked-sequence {
                      tunnel: w891 -> [_ w898 _]
                      tunnel: [_ w897 _] -> w890
                      tunnel: [_ w896 _] -> w889
                      frame #0 {
                        n218 = property on="RAM" class="Bool (strict)"("Blinking"=TRUE) -> ()  [unwired: 2 in, 2 out]
                        n219 = property on="ON" class="Bool (strict)"("Blinking"=FALSE) -> ()  [unwired: 2 in, 2 out]
                      }
                      frame #1 {
                        n220 = for {
                          N: 6 -> [_]
                          tunnel: w898 -> [w902]
                          tunnel: [w901] -> w897
                          tunnel: [w900] -> w896
                          i -> [w904]
                          n221 = flat-sequence {
                            tunnel: w904 -> [w906]
                            tunnel: [w907] -> w903
                            tunnel: w903 -> [w926]
                            tunnel: [w927] -> w905
                            tunnel: w902 -> [w930]
                            tunnel: [w929] -> w900
                            tunnel: [w928] -> w901
                            tunnel: w905 -> [w936]
                            tunnel: w904 -> [w935]
                            frame #0 {
                              n222 = case shown="0, Default" w906 {
                                tunnel: [w910 w914 w918 "*R27" "*R28" w924] -> w907
                                frame 0, Default {
                                n223 = local read "RAM"() -> (w911:bool)
                                n224 = Select(t="*G17", s=w911, f="*R17") -> (s? t:f=w910:string)
                                }
                                frame 1 {
                                n225 = local read "RAM"() -> (w915:bool)
                                n226 = Select(t="*G18", s=w915, f="*R18") -> (s? t:f=w914:string)
                                }
                                frame 2 {
                                n227 = local read "RAM"() -> (w919:bool)
                                n228 = Select(t="*G19", s=w919, f="*R19") -> (s? t:f=w918:string)
                                }
                                frame 3 {
                                }
                                frame 4 {
                                }
                                frame 5 {
                                n229 = local read "RAM"() -> (w925:bool)
                                n230 = Select(t="*G01", s=w925, f="*R01") -> (s? t:f=w924:string)
                                }
                              }
                            }
                            frame #1 {
                              n231 = Unbundle(w930) -> ("VISA resource name out"=w934:refnum<visa-resource-name>, "error out"=w932:errorcluster, "Delay (ms)"=w933:u32, "Write/\nRead"=w931:bool)
                              n232 = call "I3252_Comm_Interface.vi"("VISA resource name in"=w934, "error in"=w932, "Delay (ms)"=w933, "Write"=w931, "String to Write"=w926, "Read"=w931) -> ("VISA resource name out"=w928:refnum<visa-resource-name>, "error out"=w929:errorcluster, "Read String"=w927:string)  [unwired: 2 in]
                            }
                            frame #2 {
                              n233 = case shown="0, Default" w935 {
                                tunnel: w936 -> [w938 w942 w946 w950 w954 w958]
                                frame 0, Default {
                                n234 = String Subset(string=w938, offset (0)=3) -> (substring=w939:string)  [unwired: 1 in]
                                n235 = Hexadecimal String To Number(string=w939) -> (number=w937:u32)  [unwired: 2 in, 1 out]
                                n236 = local write "P (PB1) Sollwert"(w937) -> ()
                                n237 = local write "P (PB1) Istwert"(w937) -> ()
                                }
                                frame 1 {
                                n238 = String Subset(string=w942, offset (0)=3) -> (substring=w943:string)  [unwired: 1 in]
                                n239 = Hexadecimal String To Number(string=w943) -> (number=w941:u32)  [unwired: 2 in, 1 out]
                                n240 = local write "I ( Reset1) Sollwert"(w941) -> ()
                                n241 = local write "I ( Reset1) Istwert"(w941) -> ()
                                }
                                frame 2 {
                                n242 = String Subset(string=w946, offset (0)=3) -> (substring=w947:string)  [unwired: 1 in]
                                n243 = Hexadecimal String To Number(string=w947) -> (number=w945:u32)  [unwired: 2 in, 1 out]
                                n244 = local write "D (Rate) IstWert"(w945) -> ()
                                n245 = local write "D (Rate) Sollwert"(w945) -> ()
                                }
                                frame 3 {
                                n246 = String Subset(string=w950, offset (0)=3) -> (substring=w951:string)  [unwired: 1 in]
                                n247 = Hexadecimal String To Number(string=w951) -> (number=w949:u32)  [unwired: 2 in, 1 out]
                                n248 = local write "% LOW Istwert"(w949) -> ()
                                n249 = local write "% LOW Sollwert"(w949) -> ()
                                }
                                frame 4 {
                                n250 = String Subset(string=w954, offset (0)=3) -> (substring=w955:string)  [unwired: 1 in]
                                n251 = Hexadecimal String To Number(string=w955) -> (number=w953:u32)  [unwired: 2 in, 1 out]
                                n252 = local write "% HIGH Istwert"(w953) -> ()
                                n253 = local write "% High Sollwert"(w953) -> ()
                                }
                                frame 5 {
                                n254 = call "I3252_Edit_Setpoint.vi"("Read String"=w958) -> ("Setpoint is"=w957:dbl)
                                n255 = local write "SP 1 is (°C)"(w957) -> ()
                                }
                              }
                            }
                          }
                        }
                      }
                      frame #2 {
                        n256 = property on="RAM" class="Bool (strict)"("Blinking"=FALSE) -> ()  [unwired: 2 in, 2 out]
                      }
                    }
                    n257 = Not(x="RAM") -> (.not. x?=w893:bool)
                  }
                  event "Set Gauge to Zero": Value Change {
                    n258 = event-data() -> ()  [unwired: 1 in, 1 out]
                    n259 = flat-sequence {
                      tunnel: w964 -> [w969]
                      tunnel: [w969] -> w963
                      tunnel: w963 -> [w971]
                      tunnel: [w975] -> w962
                      tunnel: [w974] -> w961
                      tunnel: [w971] -> w960
                      tunnel: w962 -> [w981]
                      tunnel: w961 -> [w980]
                      tunnel: w960 -> [w976]
                      frame #0 {
                        n260 = property on="Set Gauge to Zero" class="Bool"("Blinking"=TRUE) -> ()  [unwired: 2 in, 2 out]
                      }
                      frame #1 {
                        w972 = 0 items=["sensor 1", "sensor 2", "test"] ("Sensor Nr.:")
                        n261 = call "DUAL GAUGE-Get Pressure,Status.vi"("Sensor Nr.:"=w972, "Referenz in"=w971) -> ("Pressure"=w975:dbl)  [unwired: 6 in, 3 out]
                        n262 = call "DUAL GAUGE-Offset display.vi"("W/R"=FALSE, "Referenz in"=w971) -> ("Sensor 1 Get"=w974:dbl)  [unwired: 6 in, 3 out]
                      }
                      frame #2 {
                        n263 = Add(x=w981, y=w980) -> (x+y=w977:dbl)
                        n264 = call "DUAL GAUGE-Offset display.vi"("W/R"=TRUE, "Sensor 1 Set"=w977, "Referenz in"=w976) -> ("Sensor 1 Get"=→"Current Offset (mbar)":dbl)  [unwired: 5 in, 3 out]
                      }
                      frame #3 {
                        n265 = property on="Set Gauge to Zero" class="Bool"("Blinking"=TRUE) -> ()  [unwired: 2 in, 2 out]
                      }
                    }
                    n266 = Unbundle(w968) -> ("VISA resource name out"=w967:refnum<visa-resource-name>, "error out"=w966:errorcluster)  [unwired: 2 out]
                  }
                  event "Write to File": Value Change {
                    n267 = event-data() -> ("NewVal"=w987:bool)  [unwired: 1 in]
                    n268 = Unbundle(w990) -> ("VISA resource name out"=w989:refnum<visa-resource-name>, "error out"=w988:errorcluster)  [unwired: 2 out]
                    n269 = local read "File Path"() -> (w983:path)
                    n270 = case shown="True" w987 {
                      tunnel: w983 -> [_ w995]
                      tunnel: "User" -> [_ w994]
                      tunnel: "Sample" -> [_ w993]
                      tunnel: [path "" ("File Path") w992] -> w984
                      frame False {
                      }
                      frame True {
                        n271 = call "Header.vi"("Sample"=w993, "User"=w994, "File Path"=w995) -> ("File Path"=w992:path)
                      }
                    }
                    n272 = local write "File Path"(w984) -> ()
                  }
                }
              }
              n273 = Bundle(cluster=w426, "VISA resource name out"=w425, "error out"=w424) -> (w423:T7)  [unwired: 2 in]
            }
            frame #2 {
            }
            frame #3 {
              (unwired) "Daniel Schuster (geb. 20.03.1988)"
              n274 = node-c288(w1023) -> (w1025:T3)  [unwired: 2 in]
              n275 = timed-sequence {
                timing: w1025 -> [_]
                timing-out: [_] -> w1024
                tunnel: [w1086] -> w1027
                tunnel: [w1085] -> w1026
                tunnel: w1022 -> [w1084]
                tunnel: w1021 -> [w1083]
                tunnel: w1020 -> [w1082]
                n276 = timed-flat-sequence {
                  tunnel: [w1091] -> w1086
                  tunnel: [w1090] -> w1085
                  tunnel: w1084 -> [w1089]
                  tunnel: w1083 -> [w1088]
                  tunnel: w1082 -> [w1087]
                  n277 = node-c288() -> ()  [unwired: 1 in, 1 out]
                  n278 = case shown="True" "RUN Keithley Measurement" {
                    tunnel: w1089 -> [_ w1099]
                    tunnel: [w1094 w1098] -> w1091
                    tunnel: [w1093 w1097] -> w1090
                    tunnel: w1088 -> [w1094 w1096]
                    tunnel: w1087 -> [w1093 w1095]
                    frame False {
                    }
                    frame True {
                      n279 = flat-sequence {
                        tunnel: [w1108] -> w1103
                        tunnel: [w1107] -> w1102
                        tunnel: w1096 -> [w1105]
                        tunnel: w1095 -> [w1104]
                        tunnel: w1103 -> [w1111]
                        tunnel: [w1111] -> w1101
                        tunnel: w1102 -> [w1110]
                        tunnel: [w1110] -> w1100
                        tunnel: w1099 -> [w1109]
                        tunnel: w1101 -> [w1115]
                        tunnel: w1100 -> [w1114]
                        tunnel: [w1113] -> w1097
                        tunnel: [w1112] -> w1098
                        frame #0 {
                          n280 = VISA Write(VISA resource name=w1105, write buffer="meas?\n" ("write buffer 2"), error in (no error)=w1104) -> (VISA resource name out=w1108:refnum<visa-resource-name>, error out=w1107:errorcluster)  [unwired: 1 out]
                        }
                        frame #1 {
                          n281 = Wait (ms)(milliseconds to wait=w1109) -> ()  [unwired: 1 out]
                        }
                        frame #2 {
                          n282 = property class="Instr"(reference=w1115, error in=w1114) -> (reference out=w1117:refnum<visa-resource-name>, error out=w1116:errorcluster, "Bytes at Port"=w1119:u32)
                          "Bytes at Port 3" <- w1119
                          n283 = VISA Read(VISA resource name=w1117, byte count=w1119, error in (no error)=w1116) -> (VISA resource name out=w1112:refnum<visa-resource-name>, read buffer=→"read buffer 2":string, error out=w1113:errorcluster)  [unwired: 1 out]
                        }
                      }
                    }
                  }
                  n284 = node-c288() -> ()  [unwired: 1 in, 1 out]
                }
              }
              n285 = node-c288(w1059) -> (w1068:T3)  [unwired: 2 in]
              n286 = node-c288(w1074) -> (w1077:T3)  [unwired: 2 in]
              n287 = node-c288(w1064) -> (w1066:T3)  [unwired: 2 in]
              n288 = node-c288(w1073) -> (w1081:T3)  [unwired: 2 in]
              n289 = timed-sequence {
                timing: w1068 -> [_]
                timing-out: [_] -> w1067
                tunnel: w1043 -> [w1168]
                tunnel: w1042 -> [w1164]
                tunnel: [w1167] -> w1035
                tunnel: w1034 -> [w1166]
                tunnel: w1033 -> [w1165]
                tunnel: [w1163] -> w1032
                tunnel: [w1162] -> w1031
                tunnel: [w1161] -> w1030
                n290 = timed-flat-sequence {
                  tunnel: w1168 -> [w1177]
                  tunnel: [w1176] -> w1167
                  tunnel: w1166 -> [w1175]
                  tunnel: w1165 -> [w1174]
                  tunnel: w1164 -> [w1173]
                  tunnel: [w1171] -> w1163
                  tunnel: [w1170] -> w1162
                  tunnel: [w1169] -> w1161
                  n291 = node-c288() -> ()  [unwired: 1 in, 1 out]
                  n292 = case shown="True" "ON (TPG 2)" {
                    tunnel: w1173 -> [w1182 w1188]
                    tunnel: w1174 -> [w1181 w1187]
                    tunnel: [w1180 w1186] -> w1170
                    tunnel: [w1179 w1185] -> w1169
                    frame False {
                      w1183 = 0.0 ("Pressure")
                      n293 = property on="ON (TPG 2)" class="Bool (strict)"("Blinking"=FALSE) -> ()  [unwired: 2 in, 2 out]
                      n294 = Bundle("Pressure"=w1183, "Pressure"=w1183) -> (w1180:cluster{"Pressure":dbl, "Pressure":dbl})  [unwired: 1 in]
                      n295 = Bundle("TPG 2 COM"=w1182, "error out"=w1181) -> (w1179:T8)  [unwired: 1 in]
                    }
                    frame True {
                      n296 = stacked-sequence {
                        tunnel: w1188 -> [_ w1201]
                        tunnel: [_ w1197] -> w1186
                        tunnel: [_ w1193] -> w1185
                        tunnel: w1187 -> [_ w1190]
                        frame #0 {
                          n297 = property on="ON (TPG 2)" class="Bool (strict)"("Blinking"=TRUE) -> ()  [unwired: 2 in, 2 out]
                        }
                        frame #1 {
                          n298 = call "PresureGetSubVI.vi"("COM in"=w1201, "Fehler (Eingang)"=w1190) -> ("Status Gauge#1"=→"Status Gauge 2#1":i32, "Status Gauge#2"=→"Status Gauge 2#2":i32, "COM out"=w1194:refnum<visa-resource-name>, "Pressure Gauge#1"=w1195:dbl, "Pressure Gauge#2"=w1198:dbl, "Cluster (Ausgang)"=w1191:errorcluster)  [unwired: 12 in]
                          "Pressure Gauge 2#1" <- w1195
                          "Pressure Gauge 2#2" <- w1198
                          n299 = Bundle("COM out"=w1194, "Cluster (Ausgang)"=w1191) -> (w1193:T9)  [unwired: 1 in]
                          n300 = Unbundle(w1191) -> ("status"=w1192:bool, "code"=w1196:i32)  [unwired: 1 out]
                          n301 = Bundle("status"=w1192, "code"=w1196) -> ()  [unwired: 1 in, 1 out]
                          n302 = Bundle("Pressure Gauge#1"=w1195, "Pressure Gauge#2"=w1198) -> (w1197:T10)  [unwired: 1 in]
                        }
                      }
                    }
                  }
                  n303 = case shown="True" "ON (TPG 1)" {
                    tunnel: w1177 -> [w1205 w1211]
                    tunnel: [w1204 w1210] -> w1176
                    tunnel: w1175 -> [w1203 w1209]
                    tunnel: [w1202 w1208] -> w1171
                    frame False {
                      w1206 = 0.0 ("Pressure")
                      n304 = property on="ON (TPG 1)" class="Bool (strict)"("Blinking"=FALSE) -> ()  [unwired: 2 in, 2 out]
                      n305 = Bundle("Pressure"=w1206, "Pressure"=w1206) -> (w1202:cluster{"Pressure":dbl, "Pressure":dbl})  [unwired: 1 in]
                      n306 = Bundle("TPG 1 COM"=w1205, "error out"=w1203) -> (w1204:T11)  [unwired: 1 in]
                    }
                    frame True {
                      n307 = stacked-sequence {
                        tunnel: w1211 -> [_ w1224]
                        tunnel: [_ w1217] -> w1210
                        tunnel: w1209 -> [_ w1214]
                        tunnel: [_ w1213] -> w1208
                        frame #0 {
                          n308 = property on="ON (TPG 1)" class="Bool (strict)"("Blinking"=TRUE) -> ()  [unwired: 2 in, 2 out]
                        }
                        frame #1 {
                          n309 = call "PresureGetSubVI.vi"("COM in"=w1224, "Fehler (Eingang)"=w1214) -> ("Status Gauge#1"=→"Status Gauge 1#1":i32, "Status Gauge#2"=→"Status Gauge 1#2":i32, "COM out"=w1218:refnum<visa-resource-name>, "Pressure Gauge#1"=w1219:dbl, "Pressure Gauge#2"=w1221:dbl, "Cluster (Ausgang)"=w1215:errorcluster)  [unwired: 12 in]
                          "Pressure Gauge 1#1" <- w1219
                          "Pressure Gauge 1#2" <- w1221
                          n310 = Bundle("COM out"=w1218, "Cluster (Ausgang)"=w1215) -> (w1217:T9)  [unwired: 1 in]
                          n311 = Unbundle(w1215) -> ("status"=w1216:bool, "code"=w1220:i32)  [unwired: 1 out]
                          n312 = Bundle("status"=w1216, "code"=w1220) -> ()  [unwired: 1 in, 1 out]
                          n313 = Bundle("Pressure Gauge#1"=w1219, "Pressure Gauge#2"=w1221) -> (w1213:T10)  [unwired: 1 in]
                        }
                      }
                    }
                  }
                  n314 = node-c288() -> ()  [unwired: 1 in, 1 out]
                }
              }
              n315 = timed-sequence {
                timing: w1077 -> [_]
                timing-out: [_] -> w1076
                tunnel: w1075 -> [w1234]
                tunnel: [w1233] -> w1070
                tunnel: [w1232] -> w1069
                tunnel: [w1231] -> w1056
                n316 = timed-flat-sequence {
                  tunnel: w1234 -> [w1238]
                  tunnel: [w1237] -> w1233
                  tunnel: [w1236] -> w1232
                  tunnel: [w1235] -> w1231
                  n317 = node-c288() -> ()  [unwired: 1 in, 1 out]
                  n318 = case shown="True" "ON" {
                    tunnel: w1238 -> [w1242 w1247]
                    tunnel: [w1241 w1246] -> w1237
                    tunnel: [w1240 w1245] -> w1236
                    tunnel: [_ w1244] -> w1235
                    frame False {
                      n319 = Unbundle(w1242) -> ("VISA resource name out"=w1241:refnum<visa-resource-name>, "error out"=w1240:errorcluster)  [unwired: 2 out]
                      n320 = property on="ON" class="Bool (strict)"("Blinking"=FALSE) -> ()  [unwired: 2 in, 2 out]
                    }
                    frame True {
                      n321 = stacked-sequence {
                        tunnel: w1247 -> [_ w1252]
                        tunnel: [_ w1251] -> w1246
                        tunnel: [_ w1250] -> w1245
                        tunnel: [_ w1249] -> w1244
                        frame #0 {
                          n322 = property on="ON" class="Bool (strict)"("Blinking"=TRUE) -> ()  [unwired: 2 in, 2 out]
                        }
                        frame #1 {
                          n323 = Unbundle(w1252) -> ("VISA resource name out"=w1256:refnum<visa-resource-name>, "error out"=w1254:errorcluster, "Delay (ms)"=w1255:u32, "Write/\nRead"=w1253:bool)
                          n324 = call "I3252_Comm_Interface.vi"("VISA resource name in"=w1256, "error in"=w1254, "Delay (ms)"=w1255, "Write"=w1253, "String to Write"="*V01", "Read"=w1253) -> ("VISA resource name out"=w1251:refnum<visa-resource-name>, "error out"=w1250:errorcluster, "Read String"=w1249:string)  [unwired: 2 in]
                        }
                      }
                    }
                  }
                  n325 = node-c288() -> ()  [unwired: 1 in, 1 out]
                }
              }
              n326 = timed-sequence {
                timing: w1066 -> [_]
                timing-out: [_] -> w1065
                tunnel: w1063 -> [w1130]
                tunnel: w1062 -> [w1129]
                tunnel: [w1128] -> w1060
                tunnel: [w1127] -> w1061
                tunnel: [w1126] -> w1057
                n327 = timed-flat-sequence {
                  tunnel: w1130 -> [w1135]
                  tunnel: w1129 -> [w1134]
                  tunnel: [w1133] -> w1128
                  tunnel: [w1132] -> w1127
                  tunnel: [w1131] -> w1126
                  n328 = node-c288() -> ()  [unwired: 1 in, 1 out]
                  n329 = case shown="False" "ON" {
                    tunnel: w1135 -> [w1139 w1145]
                    tunnel: w1134 -> [w1140 w1144]
                    tunnel: [w1139 w1143] -> w1133
                    tunnel: [w1140 w1142] -> w1132
                    tunnel: [0.0 ("Reading") w1141] -> w1131
                    frame False {
                      n330 = property on="ON" class="Bool (strict)"("Blinking"=FALSE) -> ()  [unwired: 2 in, 2 out]
                    }
                    frame True {
                      n331 = stacked-sequence {
                        tunnel: w1145 -> [_ w1152]
                        tunnel: w1144 -> [_ w1151]
                        tunnel: [_ w1150] -> w1143
                        tunnel: [_ w1149] -> w1142
                        tunnel: [_ w1147] -> w1141
                        frame #0 {
                          n332 = property on="ON" class="Bool (strict)"("Blinking"=TRUE) -> ()  [unwired: 2 in, 2 out]
                        }
                        frame #1 {
                          n333 = call "VC840_Read.vi"("error in (no error)"=w1151, "VISA resource name"=w1152) -> ("error out"=w1149:errorcluster, "Unit"=→"Unit 2":string, "Reading"=w1147:dbl, "VISA resource name out"=w1150:refnum<visa-resource-name>, "Status"=→"Status 2":T2, "Mode"=→"Mode 2":enum16{"?", "Diode", "Beep", "DC", "AC"})  [unwired: 4 out]
                          "Reading 2" <- w1147
                        }
                      }
                    }
                  }
                  n334 = node-c288() -> ()  [unwired: 1 in, 1 out]
                }
              }
              n335 = timed-sequence {
                timing: w1081 -> [_]
                timing-out: [_] -> w1080
                tunnel: w1079 -> [w1268]
                tunnel: w1078 -> [w1267]
                tunnel: [w1266] -> w1072
                tunnel: [w1265] -> w1071
                tunnel: [w1264] -> w1058
                n336 = timed-flat-sequence {
                  tunnel: w1268 -> [w1273]
                  tunnel: w1267 -> [w1272]
                  tunnel: [w1271] -> w1266
                  tunnel: [w1270] -> w1265
                  tunnel: [w1269] -> w1264
                  n337 = node-c288() -> ()  [unwired: 1 in, 1 out]
                  n338 = case shown="True" "ON" {
                    tunnel: w1273 -> [w1277 w1283]
                    tunnel: w1272 -> [w1278 w1282]
                    tunnel: [w1277 w1281] -> w1271
                    tunnel: [w1278 w1280] -> w1270
                    tunnel: [0.0 ("Reading") w1279] -> w1269
                    frame False {
                      n339 = property on="ON" class="Bool (strict)"("Blinking"=FALSE) -> ()  [unwired: 2 in, 2 out]
                    }
                    frame True {
                      n340 = stacked-sequence {
                        tunnel: w1283 -> [_ w1290]
                        tunnel: w1282 -> [_ w1289]
                        tunnel: [_ w1288] -> w1281
                        tunnel: [_ w1287] -> w1280
                        tunnel: [_ w1285] -> w1279
                        frame #0 {
                          n341 = property on="ON" class="Bool (strict)"("Blinking"=TRUE) -> ()  [unwired: 2 in, 2 out]
                        }
                        frame #1 {
                          n342 = call "VC840_Read.vi"("error in (no error)"=w1289, "VISA resource name"=w1290) -> ("error out"=w1287:errorcluster, "Unit"=→"Unit 1":string, "Reading"=w1285:dbl, "VISA resource name out"=w1288:refnum<visa-resource-name>, "Status"=→"Status 1":T2, "Mode"=→"Mode 1":enum16{"?", "Diode", "Beep", "DC", "AC"})  [unwired: 4 out]
                          "Reading 1" <- w1285
                        }
                      }
                    }
                  }
                  n343 = node-c288() -> ()  [unwired: 1 in, 1 out]
                }
              }
              n344 = Tick Count (ms)() -> (millisecond timer value=w1044:u32)
              n345 = Subtract(x=w1044, y=w1049) -> (x-y=w1048:u32)
              n346 = Divide(x=w1048, y=u32 1000) -> (x/y=w1046:dbl)
              n347 = node-c288(w1080) -> ()  [unwired: 1 out]
              n348 = node-c288(w1065) -> ()  [unwired: 1 out]
              n349 = node-c288(w1076) -> ()  [unwired: 1 out]
              n350 = To Double Precision Float(number=w1046) -> (double precision float=w1050:dbl)
              "current time (s)" <- w1050
              n351 = node-c288(w1067) -> ()  [unwired: 1 out]
              n352 = Unbundle(w1031) -> ("Pressure Gauge#1"=w1028:dbl, "Pressure Gauge#2"=w1029:dbl)
              "Pressure Gauge 2#2" <- w1029
              "Pressure Gauge 2#1" <- w1028
              n353 = Unbundle(w1032) -> ("Pressure Gauge#1"=w1041:dbl, "Pressure Gauge#2"=w1036:dbl)
              "Pressure Gauge 1#1" <- w1041
              "Pressure Gauge 1#2" <- w1036
              n354 = node-c288(w1024) -> ()  [unwired: 1 out]
            }
            frame #4 {
              n355 = Build Array (concatenate)(w1312, w1316) -> (w1311:dbl[])
              n356 = Build Array (concatenate)(w1315, w1317) -> (w1310:dbl[])
              n357 = Build Array (concatenate)(w1313, w1304) -> (w1308:dbl[])
              n358 = Build Array (concatenate)(w1314, w1305) -> (w1309:dbl[])
              n359 = Greater?(x=w1336, y="Pressure Limit (mbar)") -> (0:w1339:bool)
              n360 = case shown="False" w1339 {
                frame False {
                  n361 = property on="Standby" class="Bool (strict)"("DisabledEnum"=T6."Enabled" ("Disabled")) -> ()  [unwired: 2 in, 2 out]
                }
                frame True {
                  n362 = property on="Standby" class="Bool (strict)"("Val(Sgnl)"=TRUE ("Standby"), "DisabledEnum"=T6."Disabled" ("Disabled")) -> ()  [unwired: 2 in, 2 out]
                }
              }
              n363 = call "Resistivity_Calculation.vi"("Reading 1 (V)"=w1329, "Constant"="4PP constant", "Thickness (nm)"="Thickness (nm)", "Reading 2 (A)"=w1337) -> ("Resivtivity (Ohm*cm)"=w1321:dbl, "Current"=w1322:dbl, "Voltage"=w1323:dbl)
              "Resistivity (Ohm*cm)" <- w1321
              "Voltage (V)" <- w1323
              "Current (A)" <- w1322
              n364 = call "I3252_Edit_Temperature.vi"("Temp. String"=w1338) -> ("Temp. (°C)"=w1332:dbl)
              "(°C)" <- w1332
              n365 = Build Array (concatenate)(w1334, w1335) -> (w1331:dbl[])
              n366 = Build Array (concatenate)(w1333, w1332) -> (w1319:dbl[])
              n367 = Build Array (concatenate)(w1330, w1323) -> (w1328:dbl[])
              n368 = Build Array (concatenate)(w1327, w1322) -> (w1325:dbl[])
              n369 = Build Array (concatenate)(w1326, w1321) -> (w1324:dbl[])
              n370 = Build Array(w1323, w1322, w1321) -> (w1320:dbl[])
            }
            frame #5 {
              n371 = Bundle(w1369, w1368) -> (→"Main Chamber (PG-1)":cluster{dbl[], dbl[]})  [unwired: 1 in]
              n372 = Bundle(w1369, w1367) -> (→"Loadlock (PG-3)":cluster{dbl[], dbl[]})  [unwired: 1 in]
              n373 = Bundle(w1369, w1366) -> (→"Pirani (VVP1 Scroll)":cluster{dbl[], dbl[]})  [unwired: 1 in]
              n374 = Bundle(w1369, w1365) -> (→"Pressure OpenPort":cluster{dbl[], dbl[]})  [unwired: 1 in]
              n375 = Bundle(w1369, w1375) -> (→"Sample holder (Type-K Thermocouple)":cluster{dbl[], dbl[]})  [unwired: 1 in]
              n376 = Bundle(w1369, w1377) -> (→"Voltage":cluster{dbl[], dbl[]})  [unwired: 1 in]
              n377 = Bundle(w1369, w1378) -> (→"Current":cluster{dbl[], dbl[]})  [unwired: 1 in]
              n378 = Bundle(w1369, w1379) -> (→"Resistivity":cluster{dbl[], dbl[]})  [unwired: 1 in]
              n379 = Build Array (concatenate)(w1374, w1384, w1383, w1373, w1360, w1357, w1355) -> (w1391:dbl[])
              "appended array" <- w1391
              n380 = call "array_to_xy-graph.vi"() -> ()  [unwired: 3 in, 1 out]
            }
            frame #6 {
              n381 = Unbundle(w1399) -> ("COM out"=w1398:refnum<visa-resource-name>, "Cluster (Ausgang)"=w1397:errorcluster)
              n382 = Unbundle(w1396) -> ("COM out"=w1395:refnum<visa-resource-name>, "Cluster (Ausgang)"=w1394:errorcluster)
              n383 = case shown="True" "Write to File" {
                tunnel: [_ w1427] -> w1413
                tunnel: "File Path" -> [_ w1425]
                tunnel: w1406 -> [_ w1423]
                frame False {
                  n384 = property on="Write to File" class="Bool (strict)"("Blinking"=FALSE) -> ()  [unwired: 2 in, 2 out]
                }
                frame True {
                  n385 = flat-sequence {
                    tunnel: [w1429] -> w1426
                    tunnel: w1425 -> [w1429]
                    tunnel: [w1428] -> w1424
                    tunnel: w1423 -> [w1428]
                    tunnel: [w1434] -> w1427
                    tunnel: w1426 -> [w1433]
                    tunnel: w1424 -> [w1432]
                    frame #0 {
                      n386 = property on="Write to File" class="Bool (strict)"("Blinking"=TRUE) -> ()  [unwired: 2 in, 2 out]
                    }
                    frame #1 {
                      n387 = call-poly <vilib>:"Write To Spreadsheet File.vi"("format (%.3f)"="%g", "append to file? (new file:F)"=TRUE ("transpose? (no:F)"), "1D data"=w1432, "file path (dialog if empty)"=w1433) -> ("new file path (Not A Path if cancelled)"=w1434:path)  [unwired: 4 in]
                    }
                  }
                }
              }
              n388 = Merge Errors(w1418, w1417, w1415, w1397, w1394) -> (w1416:errorcluster)
              n389 = call <vilib>:"Simple Error Handler.vi"("error in (no error)"=w1416) -> ("error?"=w1400:bool)  [unwired: 4 in, 4 out]
              n390 = local write "File Path"(w1413) -> ()
            }
            frame #7 {
              w1453 = u32 1000 ("y")
              n391 = Tick Count (ms)() -> (millisecond timer value=w1455:u32)
              n392 = Subtract(x=w1455, y=w1454) -> (x-y=w1456:u32)
              n393 = VISA Flush I/O Buffer(VISA resource name=w1448, error in (no error)=w1447) -> (VISA resource name out=w1445:refnum<visa-resource-name>, error out=w1446:errorcluster)  [unwired: 1 in]
              n394 = VISA Flush I/O Buffer(VISA resource name=w1441, error in (no error)=w1440) -> (VISA resource name out=w1444:refnum<visa-resource-name>, error out=w1443:errorcluster)  [unwired: 1 in]
              n395 = Divide(x=w1456, y=w1453) -> (x/y=w1439:ext)
              "loop time (s)" <- w1439
              n396 = Subtract(x="Intervall (s)", y=w1439) -> (x-y=w1438:ext)
              n397 = Multiply(x=w1438, y=w1453) -> (x*y=w1458:ext)
              n398 = Wait (ms)(milliseconds to wait=w1458) -> ()  [unwired: 1 out]
              n399 = Bundle("COM out"=w1445, "error out"=w1446, "COM out"=w1444, "error out"=w1443) -> (w1442:T12)  [unwired: 1 in]
            }
            frame #8 {
              n400 = Tick Count (ms)() -> (millisecond timer value=w1480:u32)
              n401 = Subtract(x=w1480, y=w1478) -> (x-y=w1479:u32)
              n402 = Divide(x=w1479, y=w1477) -> (x/y=→"data logger intervall (s)":dbl)
            }
          }
          n403 = Exclusive Or(1:"stop", 2:w183) -> (0:w184:bool)
        }
      }
      frame #4 {
        n404 = call "VC840_Close.vi"("error in (no error)"=w1502, "VISA resource name"=w1503) -> ("error out"=w1511:errorcluster)  [unwired: 9 in]
        n405 = call "VC840_Close.vi"("error in (no error)"=w1504, "VISA resource name"=w1505) -> ("error out"=w1509:errorcluster)  [unwired: 9 in]
        n406 = VISA Close(VISA resource name=w1507, error in (no error)=w1506) -> (error out=w1508:errorcluster)
        n407 = VISA Close(VISA resource name=w1494, error in (no error)=w1493) -> (error out=→"error out":errorcluster)
        n408 = Unbundle(w1500) -> ("COM out"=w1499:refnum<visa-resource-name>, "error out"=w1498:errorcluster, "COM out"=w1496:refnum<visa-resource-name>, "error out"=w1497:errorcluster)
        n409 = VISA Close(VISA resource name=w1499, error in (no error)=w1498) -> ()  [unwired: 1 out]
        n410 = VISA Close(VISA resource name=w1496, error in (no error)=w1497) -> ()  [unwired: 1 out]
        n411 = Merge Errors(w1508, w1509, w1511) -> (w1510:errorcluster)
        n412 = call <vilib>:"Simple Error Handler.vi"("error in (no error)"=w1510) -> ("error?"=w1501:bool)  [unwired: 1 in, 7 out]
        n413 = Stop(stop? (T)=w1501) -> ()
      }
    }
  }
